vi "Find interstitial position.vi"(8 "Sublattice Index":i32, 9 "Interstitial Type":T3(ring), 10 "Suggested Location":dbl[](array[numeric])=[0.001, 6.609982847865, 13.218965695729999], 11 "Input Structure":T1={"Structure Name"="Gamma8_64atom Expanded to Box", "Lattice vector a"=[13.21796569573, 0.0, 0.0], "Lattice vector b"=[0.0, 13.21796569573, 0.0], "Lattice vector c"=[0.0, 0.0, 13.21796569573], "Atoms Array"=[{"Atom Name"="Cd", "Positions (Direct)"=array171x3[513 elements], "Positions (Cartesian)"=array171x3[513 elements]}, {"Atom Name"="Te", "Positions (Direct)"=array256x3[768 elements], "Positions (Cartesian)"=array256x3[768 elements]}], "# of atoms"=427}) -> (2 "Actual Position":dbl[](array[numeric])=[-1.6522457119662501, 8.261228559831249, 14.87021140769625])   [LabVIEW 2010]
uses:
  <vilib>/Analysis/_algsub.llb/Real Vector Norm.vi
  <vilib>/Analysis/NI_AALPro.lvlib
panel:
  out "Array 5":dbl[][](array[numeric])=[[4.672549508441724, 4.672549508441724, 4.672549508441726, 4.673256668714749, 4.6732566687147505, 4.673256668714748, 4.6732566687147505, 4.6732566687147505, 4.67325666871475, 4.673963721996005, 4.673963721996006, 4.673963721996005, 6.608482885695166, 6.608482885695166, 6.609482885689442, 6.609482885689441, 8.093501356604872, 8.093501356604872, 8.093909635782499, 8.093909635782499, 8.093909635782499, 8.093909635782499, 8.094317894366434, 8.094317894366432, 8.094317894366434, 8.094317894366434, 8.094726132359792, 8.09472613235979, 8.094726132359792, 8.094726132359792, 8.09513434976569, 8.09513434976569, 9.345806083535642, 9.346513217063759, 9.346513217063759, 9.346513217063759, 9.34722029709599, 10.449086969335582, 10.449086969335582, 10.449086969335582, 10.449086969335582, 10.449403211455978, 10.449403211455978, 10.449403211455978, 10.449403211455978, 10.45003566698613, 10.450035666986132, 10.450035666986132, 10.450035666986132, 10.450351880397623, 10.450351880397623, 10.450351880397623, 10.450351880397623, 11.446805432839044, 11.447382783106764, 12.363472966495479, 12.363472966495479, 12.363740242180455, 12.363740242180455, 12.364007512087667, 12.364007512087667, 12.364007512087667, 12.364274776217494, 12.364274776217494, 12.364274776217494, 12.364274776217494, 12.364274776217494, 12.364274776217494, 12.364542034570308, 12.364542034570308, 12.364542034570308, 12.364809287146482, 12.364809287146482, 12.365076533946393, 12.365076533946395, 13.217465714644366, 13.218465714642937, 14.019062667548008, 14.01906266754801, 14.019298379715233, 14.019298379715234, 14.0195340879194, 14.019769792160709, 14.019769792160709, 14.019769792160709, 14.02000549243936, 14.020241188755552, 14.02024118875555, 14.020476881109484, 14.020476881109484, 14.777464099713631, 14.777911326842537, 14.777911326842537, 14.77835854043732, 14.77835854043732, 14.77880574049921, 15.499012269911264, 15.499225475026416, 15.499225475026416, 15.499651876458502, 15.4996518764585, 15.49986507277568, 16.18822746580202, 16.188635719239674, 16.18863571923967, 16.189043962382037, 16.848881792586056, 16.84907791671063, 16.84907791671063, 16.84907791671063, 16.849274038552334, 16.849274038552334, 16.84947015811125, 16.849470158111252, 16.84966627538746, 16.84966627538746, 16.849666275387456, 16.84966627538746, 16.849862390381034, 16.849862390381034, 16.850058503092065, 16.850058503092065, 16.850254613520626, 16.850254613520622, 16.850254613520622, 16.850450721666792, 18.09871464894432, 18.09889722957616, 18.099079808366156, 18.099079808366156, 18.09926238531436, 18.09926238531436, 18.099627533685634, 18.099627533685634, 18.09981010510881, 18.09981010510881, 18.09999267469042, 18.10017524243052, 18.693026373944644, 19.267644542789487, 19.267987549118388, 19.26815904999305, 19.268159049993052, 19.268159049993052, 19.268502047163004, 19.268502047163004, 19.268502047163004, 19.268673543458373, 19.26901653147011, 19.826781895141632, 19.827115228474657, 20.36976655471307, 20.369928779363836, 20.37025322478959, 20.370253224789593, 20.370253224789593, 20.37025322478959, 20.370577665047854, 20.370739883239253, 21.415397772224, 21.41555207612973, 21.41555207612973, 21.41570637892368, 23.366000113979208, 23.366141536619267, 23.366282958403378, 23.36642437933155, 23.36656579940381, 24.282817476411132, 24.28308964193794], [4.121068592009394, 4.121068592009396, 4.121603126043498, 4.1216031260434995, 4.926194072761157, 4.9261940727611595, 5.616686189952471, 5.61668618995247, 5.617078399396615, 5.6170783993966165, 6.231480198063994, 5.61629395311869, 6.789868127999895, 7.7891381166692994, 7.789138116669298, 6.789543667070974, 7.306002937376851, 6.789868127999896, 8.242671674725111, 8.242671674725113, 7.788572438092881, 7.78885528251651, 8.673281849437187, 8.673281849437188, 9.083258983078276, 8.673535843492077, 8.673535843492076, 9.475746696494848, 9.47574669649485, 9.475979181314102, 9.475979181314104, 8.67277383901172, 9.475514205971507, 10.214936166974272, 10.214936166974274, 10.904736782714235, 9.082773903193985, 9.475049207810867, 10.214504829810819, 10.21450482981082, 9.475281709743651, 9.851940884561692, 10.904130700545782, 10.904130700545783, 11.233372335394707, 11.23337233539471, 11.552853748728355, 11.552853748728355, 11.553044435475528, 11.863920576351129, 11.553044435475526, 11.863920576351127, 11.552472365791504, 12.750981632607322, 11.232587861724038, 11.5520909702636, 11.863177798874412, 12.166131809314017, 12.166312883949994, 12.750636086798133, 12.750636086798133, 12.166493955891026, 12.750808860873262, 13.033146293985183, 13.309495784375729, 13.033146293985181, 13.309495784375729, 12.750981632607324, 13.580385110031902, 13.580385110031902, 13.84597564056925, 13.84597564056925, 13.8461347468455, 13.8461347468455, 13.309164739275896, 14.36212355005444, 13.308999213638101, 13.579736219180225, 14.105785805791598, 14.105785805791598, 14.612910408786753, 14.106098155620577, 14.860058287829462, 14.86005828782946, 14.860206536460197, 14.860354783611985, 15.342414924731075, 15.342558512555073, 15.577993369656815, 14.361356583700655, 15.34198415319593, 15.341984153195932, 15.342271335563247, 15.809643929002224, 16.263861920428326, 15.341840559996374, 15.57742769107951, 15.80936523661549, 16.705207092922233, 16.705207092922233, 16.921823947786486, 16.263184639667976, 16.705075217695192, 17.13531702235606, 17.55526852148856, 16.03753681002498, 16.704679585767526, 16.704679585767526, 16.485343319120254, 17.135059891331423, 17.135059891331423, 17.346309670416233, 17.346309670416233, 17.135317022356062, 17.555017541558783, 17.76114907877112, 17.76114907877112, 17.135445586421458, 17.9650382215233, 17.76139714593035, 17.965160847856563, 17.96528347335281, 18.166760470480675, 18.366027379531886, 18.366147328557506, 17.554515570934324, 17.964547707819758, 18.36542762265253, 18.365427622652533, 18.757742113038155, 18.757742113038155, 18.757977000635638, 18.95102838555922, 18.758094443331412, 19.331462290438033, 19.518955299633447, 19.51906816366124, 19.518616703634326, 18.757389776126885, 19.33100644902812, 19.518503836996, 19.88797484568549, 19.88797484568549, 19.704328959034704, 20.250923605296144, 20.42987230947458, 20.60737402688409, 20.78346583163942, 20.250706034368534, 20.957552569971597, 20.25048846110334, 20.606946409636635, 21.301975381695218, 20.783041837533364, 20.957447452744763, 21.301975381695218, 21.641222668030355, 21.808867468755267, 21.974732126453016, 22.13985170979759, 22.303650137269525, 22.46635242197059, 23.572912488272582, 23.726912670683017, 24.182847599331026, 24.482117462115625, 24.630433555487564, 24.77750622801834, 25.358484373325638, 0.0], [4.524587386078812, 5.09231998205977, 3.874966286339239, 4.524952541816038, 5.603111553104299, 6.50496138707789, 6.070806442471428, 5.092968857408524, 5.603406425376871, 6.505215379893139, 6.07053427389457, 7.660986458166829, 8.343679408145237, 7.661417786223605, 7.29572321537556, 8.0091972635348, 6.504707384344847, 8.664306600558447, 9.273072437942245, 8.664306600558449, 8.009609840002271, 8.6644972941253, 9.563106645654948, 9.844431954236441, 8.974221394458146, 8.009816120266752, 9.844599788361915, 10.118101441398835, 9.273606952723192, 9.563452185221488, 9.562761093602722, 10.117938144059453, 10.643887253154116, 11.145043715872097, 11.145340210668671, 9.272894259501733, 10.117611541473876, 10.897043574310901, 11.144747213187577, 9.562933871189628, 10.38408395483256, 11.624472396978694, 11.856989090555045, 10.897498434718967, 11.857267782941785, 12.30912112407838, 11.624756663731397, 11.857407126678797, 12.309255352727742, 11.145340210668671, 11.857407126678797, 12.528674536829765, 13.37212106489996, 11.856710391617629, 12.308584194842918, 12.744575824396993, 13.166012172053, 12.957135069939262, 13.166137664709101, 13.774130693526065, 12.528806413271395, 13.574614140679618, 13.971034773386775, 14.16508540124641, 13.166263156169087, 13.971034773386775, 13.166388646432988, 13.971153035115119, 14.356628458710277, 14.35674354416327, 14.165318683582521, 13.971389555568704, 13.774610496418132, 14.164852115068351, 14.916285749111236, 14.16473547053853, 14.356168107672538, 14.731684587922098, 15.097754613480275, 15.45526325984557, 14.73190889806441, 15.8046869786592, 15.27771694780128, 15.63111010771154, 15.277933241115514, 15.976688369673775, 15.631321511063923, 15.805000600052866, 15.277392502088265, 15.976378118566092, 16.314543247000234, 15.976584953307304, 16.646038384911055, 16.646236898914424, 16.31444197227772, 16.481024032009135, 16.809039732075895, 17.289589961986348, 17.446769123222808, 17.44686382506795, 17.28930327050073, 17.60245096948259, 17.90993980179392, 18.212419286233594, 16.808744844283712, 17.446390310701666, 17.602169373652973, 17.44639031070167, 17.909755294839574, 18.061538320598714, 17.75676793301744, 18.361430624238494, 17.909939801793918, 18.509599424233063, 18.65650295824463, 18.361520608602852, 17.60254483375806, 18.802346633009304, 18.361700576008616, 18.65668008017071, 18.361790559050036, 18.65676864050317, 18.80252238107122, 18.509956477832805, 18.36116066849946, 18.946631698736383, 18.946718903783477, 19.37414908003062, 19.514630123374026, 19.654023014068105, 19.514799456692987, 19.792601178364315, 19.233071485218513, 20.066639715409647, 20.066722053177486, 19.792851610620946, 20.470537751643775, 19.65377081282996, 20.33657972898106, 20.470457038133002, 20.470457038133002, 20.866698509977905, 20.33682346256355, 21.126887590461724, 21.126887590461724, 21.255787812660607, 21.12712220663944, 21.25555461667795, 21.763376075120195, 21.255399151268165, 21.637347178603495, 22.13641183778336, 21.637499899717355, 21.88837740631114, 22.01274397403771, 22.38184535746878, 22.381919178146244, 22.983390678019713, 23.101934623215634, 23.219802219673422, 23.33714531380384, 24.59005058073211, 24.700885082114148, 25.139139911160846, 25.247564075565105, 25.35552460562809, 25.782397904268457, 26.202633032169903, 0.0, 0.0]]
  out "Array 4":dbl[][](array[numeric])=[[0.5476079792120737, 0.547607979212074, 0.5476079792120737, 0.5473669639053449, 0.5473669639053448, 0.547366963905345, 0.5473669639053449, 0.5473669639053448, 0.5473669639053448, 0.5474874317712398, 0.5474874317712399, 0.5474874317712396, 0.4166189217542727, 0.41661892175427284, 0.4165658301235803, 0.4165658301235802, 1.0485123471873823, 1.0485123471873823, 0.3494728260287518, 0.34947282602875185, 0.3494728260287518, 0.3494728260287518, 1.0476668985331294, 0.3494101580745812, 0.3494101580745813, 1.047666898533129, 1.0485123471873823, 1.048512347187383, 1.0485123471873823, 1.0485123471873823, 0.3494728260287518, 0.34947282602875185, 0.5474874317712397, 0.547366963905345, 0.5473669639053449, 0.5473669639053449, 0.5476079792120738, 0.4165658301235802, 0.41656583012358017, 0.4165658301235804, 0.4165658301235802, 0.4166189217542728, 0.4166189217542727, 0.4166189217542727, 0.4166189217542728, 0.41656583012358017, 0.41656583012358017, 0.4165658301235802, 0.41656583012358006, 0.41661892175427284, 0.4166189217542727, 0.4166189217542727, 0.4166189217542726, 0.3494728260287518, 1.0485123471873827, 0.5473669639053449, 0.5473669639053451, 0.5474874317712397, 0.5474874317712396, 0.5476079792120739, 0.5476079792120737, 0.5476079792120737, 0.5473669639053449, 0.5473669639053448, 0.5473669639053448, 0.5473669639053451, 0.30695887398929206, 0.5473669639053451, 0.5474874317712398, 0.5474874317712396, 0.5474874317712397, 0.5476079792120739, 0.5476079792120737, 0.30695887398929206, 0.30695887398929206, 0.4165658301235802, 0.4166189217542728, 0.3494101580745812, 0.3494101580745813, 1.0485123471873825, 1.048512347187382, 0.34947282602875185, 0.3495041726531689, 0.34950417265316897, 0.34950417265316885, 1.0485123471873818, 0.3494728260287518, 0.34947282602875185, 0.2542774918608737, 0.3495041726531689, 0.5473669639053448, 0.5476079792120739, 0.5476079792120742, 0.5474874317712396, 0.5474874317712399, 0.30695887398929206, 0.4165658301235803, 0.4166189217542727, 0.4166189217542727, 0.4165658301235802, 0.4165658301235803, 0.4166189217542727, 1.0485123471873825, 1.047666898533129, 0.3494101580745812, 0.3494728260287518, 0.3068739535103656, 0.5473669639053448, 0.5473669639053448, 0.5473669639053448, 0.5474874317712397, 0.5474874317712399, 0.5476079792120737, 0.5476079792120738, 0.5473669639053448, 0.5473669639053451, 0.30695887398929217, 0.30695887398929206, 0.3069164049386094, 0.3069164049386095, 0.5476079792120738, 0.5476079792120742, 0.30695887398929217, 0.30695887398929217, 0.306958873989292, 0.23641690930736067, 0.34937883673726944, 1.047666898533129, 1.0485123471873825, 1.048512347187382, 0.3494728260287518, 0.34947282602875185, 1.048512347187383, 1.0485123471873827, 0.3494728260287518, 0.34947282602875185, 0.2542774918608737, 0.20968219392944848, 0.3069588739892921, 0.4164597077251133, 0.41656583012358017, 0.4164597077251134, 0.4166189217542727, 0.41661892175427284, 0.41656583012358017, 0.41656583012358045, 0.2768971596369435, 0.2769127510076522, 0.22185040368770584, 0.3494728260287518, 0.254253349262326, 0.5473669639053448, 0.5474874317712397, 0.23640720642010601, 0.547366963905345, 0.5473669639053452, 0.23640720642010596, 0.23639750472741433, 0.23640720642010601, 0.34947282602875174, 0.3494101580745812, 0.2542774918608737, 0.25425334926232607, 0.3069164049386094, 0.3068739535103656, 0.23640720642010607, 0.1993015788370914, 0.19930739241282994, 0.25426541970196903, 0.18250028210459257], [0.8561932504079697, 0.8561932504079697, 0.38283173606959353, 0.38283173606959353, 0.4280318477924466, 0.4280318477924465, 0.4942735398142433, 0.49427353981424343, 0.4941239710797636, 0.4941239710797636, 0.3494865422516429, 0.4942236684792082, 0.8561932504079699, 0.49412397107976336, 0.49412397107976347, 0.8559341113720182, 2309.4010767618342, 0.38280856217615494, 0.6053284338785394, 0.6053284338785391, 0.49422366847920796, 0.4940741450001373, 0.38283173606959353, 0.38283173606959353, 0.4280318477924465, 0.855675207490044, 0.8556752074900444, 0.4941239710797636, 0.49412397107976347, 0.4941738122369185, 0.4941738122369186, 0.8559341113720185, 0.4940741450001371, 0.38283173606959353, 0.38283173606959353, 0.4941738122369186, 0.4279670777316935, 0.4941738122369187, 0.8559341113720187, 0.8559341113720187, 0.49422366847920807, 0.34945128322800595, 0.4942236684792083, 0.49422366847920807, 0.6051452780610137, 0.6051452780610137, 0.3827622270115112, 0.3827622270115112, 0.8559341113720186, 0.4279670777316935, 0.8559341113720186, 0.4279670777316935, 0.38280856217615494, 0.8556752074900443, 0.6051452780610139, 0.8556752074900441, 0.42796707773169335, 0.49417381223691836, 0.49422366847920796, 0.38280856217615494, 0.38280856217615494, 0.4940741450001373, 0.38283173606959353, 0.30264132246286574, 0.4940741450001373, 0.30264132246286574, 0.4940741450001374, 0.855675207490044, 0.6051452780610139, 0.6051452780610139, 0.8559341113720187, 0.8559341113720182, 0.38280856217615494, 0.38280856217615494, 0.4941738122369187, 0.4941738122369186, 0.4941239710797636, 0.6051452780610138, 0.4279670777316935, 0.4279670777316935, 0.349451283228006, 0.4280318477924465, 0.38283173606959353, 0.38283173606959353, 0.3827622270115112, 0.8559341113720186, 0.4941738122369187, 0.4942236684792083, 0.6053284338785394, 0.49412397107976347, 0.4942236684792083, 0.4942236684792082, 0.49412397107976336, 0.3827622270115112, 0.4942236684792083, 0.49417381223691836, 0.6053284338785391, 0.38280856217615494, 0.8556752074900441, 0.8556752074900447, 2309.4010767618342, 0.4941738122369185, 0.38283173606959353, 0.4940741450001373, 0.8559341113720189, 0.4279023370651891, 0.3827622270115112, 0.3827622270115112, 0.349416034873861, 0.4941738122369187, 0.4941738122369187, 0.6053284338785394, 0.6053284338785394, 0.4942735398142433, 0.38283173606959353, 0.4280318477924466, 0.4280318477924465, 0.4941239710797636, 0.4941239710797636, 0.4279670777316935, 0.4941738122369187, 0.49422366847920807, 0.349451283228006, 0.8561932504079697, 0.38283173606959353, 0.38273906573776, 0.4941239710797636, 0.8559341113720189, 0.8559341113720185, 0.49422366847920807, 0.4942236684792082, 0.49412397107976347, 0.6051452780610139, 0.49417381223691836, 0.4279670777316935, 0.49422366847920807, 0.3235406796961882, 0.49427353981424343, 0.32348473632136465, 0.4279670777316935, 0.49422366847920807, 0.8561932504079699, 0.8561932504079699, 0.34948654225164283, 0.4941239710797636, 0.6051452780610138, 0.8559341113720187, 0.4280318477924465, 0.4942236684792082, 0.4941239710797636, 0.4941239710797636, 0.8559341113720185, 0.38283173606959353, 0.4280318477924464, 0.4940741450001373, 0.38283173606959353, 0.4941738122369185, 0.6053284338785391, 0.8561932504079699, 0.4280318477924465, 0.49427353981424343, 0.3494865422516429, 0.4941738122369187, 0.34945128322800595, 0.4942735398142433, 0.3827622270115112, 0.42796707773169335, 0.49422366847920807, 0.32355467007556094, 0.0], [0.5115804251230851, 0.5824808304777034, 0.33219352288401144, 0.5114389056756381, 0.3940200961906628, 0.4615602383379139, 0.4238058809752943, 0.5823241605883408, 0.3939554262004827, 0.46145629586343273, 0.4237857592774801, 0.6944091253052345, 0.4614562958634326, 0.694143717868172, 0.5824285931318084, 0.912579492565525, 0.33218383231913956, 0.5115804251230849, 0.6944091253052346, 0.5115804251230851, 0.4237053011371849, 0.5114389056756379, 0.4238058809752943, 0.46156023833791365, 0.5823241605883406, 0.9121779329760806, 0.46145629586343256, 0.34947596486447613, 0.6942321531975371, 0.42374552447850033, 0.9125794925655242, 0.5114389056756379, 0.3940200961906628, 0.46156023833791365, 0.46148227489852917, 0.3939877572149216, 0.5115450342478336, 0.9125794925655255, 1.7482263996378062, 0.42378575927747997, 0.3697306291319899, 0.5824808304777032, 0.6944091253052349, 0.9121779329760806, 0.6941437178681721, 0.46145629586343256, 0.5823241605883405, 0.6942321531975371, 0.46148227489852917, 1.746815611858634, 0.6942321531975371, 0.5115804251230848, 0.46145629586343256, 0.6942321531975368, 1.7468156118586362, 0.5824285931318085, 0.9125794925655252, 0.39400392570742504, 0.42378575927748025, 0.5824808304777033, 0.5114389056756379, 0.5114389056756378, 0.3940200961906627, 0.42380588097529426, 0.4237053011371851, 0.3940200961906629, 0.9121779329760801, 0.3939554262004827, 0.4614562958634326, 0.4614822748985293, 0.4237455244785002, 0.3939877572149216, 0.5824285931318082, 0.912579492565525, 0.694232153197537, 0.9123786464948287, 1.7468156118586369, 0.5824285931318082, 0.9125794925655252, 0.511580425123085, 0.5822719653781748, 0.39402009619066275, 0.33219352288401144, 0.5823241605883405, 1.746815611858634, 0.4237455244785004, 0.5824285931318082, 0.3939877572149215, 1.7468156118586322, 0.42378575927748013, 0.511580425123085, 0.91217793297608, 0.3939554262004827, 0.3939877572149216, 0.5115450342478336, 0.3697306291319898, 0.4237857592774801, 0.5823241605883407, 0.6941437178681721, 0.6942321531975367, 0.5824285931318082, 0.4237053011371851, 0.5114389056756379, 0.6942321531975366, 0.9121779329760806, 0.6942321531975374, 0.9123786464948292, 0.6942321531975371, 0.5115450342478336, 0.5824285931318088, 0.33218383231913956, 0.4237857592774801, 0.5114389056756378, 0.33219352288401144, 0.5114389056756381, 0.4237053011371849, 0.9121779329760801, 0.5823241605883409, 0.912378646494829, 0.511509650716535, 0.9125794925655255, 0.5115450342478336, 0.5824285931318084, 0.33218383231913956, 0.9121779329760811, 0.6942321531975372, 0.39398775721492163, 0.5115450342478336, 0.36973062913199, 0.39400392570742504, 0.5823241605883406, 0.42372541137597447, 1.7468156118586353, 0.5115096507165352, 0.5115450342478337, 0.42378575927748025, 0.4237053011371851, 0.6941437178681722, 0.39398775721492146, 0.4237857592774801, 0.4237857592774801, 0.36973062913198984, 0.6941437178681722, 0.42372541137597447, 0.9121779329760803, 1.7468156118586347, 0.42378575927748013, 0.3321838323191395, 0.9121779329760801, 0.4614822748985293, 0.3939877572149215, 0.582271965378175, 0.3940200961906627, 0.3321935228840115, 0.511438905675638, 0.9123786464948292, 0.912579492565525, 0.4237857592774801, 0.3321935228840115, 0.5114389056756382, 0.582324160588341, 0.3939877572149215, 0.4237857592774801, 0.39402009619066275, 0.9121779329760809, 1.7468156118586369, 0.4237857592774801, 0.6941437178681724, 0.0, 0.0]]
  out "Array 3":dbl[][](array[numeric])=[[1.9547268638345616, 2.8620737470709985, 3.5435417267010227, 4.113946207379072, 4.114267491346153, 4.614370902468288, 4.614657345750077, 5.065859043343244, 5.479794675188183, 5.864811600602199, 6.226064610883467, 7.202091391883803], [1.7167946955093463, 3.418443867660097, 3.418443867660097, 4.006367470857006, 4.006367470857007, 4.519014199249397, 4.978625429595594, 4.978625429595595, 4.978890916796135, 5.789856822486257, 5.789856822486257, 6.500831983269877], [3.0102934919328925, 3.010732552172754, 3.0107325521727546, 3.6646599209082016, 3.6646599209082025, 3.665020590535618, 5.151307815891239, 5.5588842449956095, 5.55888424499561, 6.955045345834196, 6.955045345834196, 6.955235391828881], [1.955267753201033, 2.861519495286735, 3.5434671227829164, 4.113881947574676, 4.114203236559899, 4.614600058516157, 4.614600058516158, 5.065545926675186, 5.864766524929215, 6.567436124440425, 6.891957826114611, 7.499163761830803], [2.5379416168562856, 2.5384623778402253, 3.2881083729171117, 3.8957513405305857, 4.420943783354774, 4.421242758402029, 4.421242758402029, 4.890052081923117, 5.713872611512734, 6.084094480605371, 6.084311731171563, 6.433045241351105], [2.166564441514756, 3.010732552172755, 3.010732552172756, 3.665020590535619, 4.708021154645086, 4.708021154645086, 5.151051215132988, 5.151051215132988, 5.15130781589124, 5.5588842449956095, 5.55888424499561, 5.938998490548465], [2.3595708433746223, 2.360130962053328, 3.7823205859257243, 3.782320585925725, 4.3210150254211985, 4.321015025421199, 5.235160141446535, 5.235160141446536, 5.235412619816098, 6.011874297027946, 6.011874297027946, 6.6993288479577675], [1.7172565860734128, 3.4179024921650596, 3.4182891976963075, 4.0062354991045535, 4.006565420335059, 4.518897199069925, 4.9785192307512744, 4.9785192307512744, 6.500547318827066, 6.500547318827066, 7.14092755186499, 7.141112650989596], [2.5383582341904414, 2.5383582341904423, 3.2876259459191286, 3.896022764532719, 4.420883985919037, 4.420883985919037, 4.421182965009993, 5.713826345100761, 5.713826345100762, 6.433209615097385, 6.763978695041821, 6.763978695041822], [2.1670524575439933, 3.0102056722001067, 3.0106447452472453, 3.6649484594496307, 4.707965003476324, 4.708245752623474, 5.150999893447406, 5.150999893447408, 5.938731409903124, 5.938731409903126, 6.295744291766251, 6.295954239068649], [2.3596828777468075, 3.152137165776393, 3.152556471343213, 3.7820410019202884, 3.7823904786980087, 4.32138208929536, 4.799954686961217, 5.235463114028928, 5.636958031913642, 6.364827311893895, 6.699171003830835, 6.6993683084084115], [1.4400732414920958, 3.288188770535453, 3.8961584694430518, 3.8961584694430518, 4.421003579981707, 4.421003579981707, 4.890106142257899, 4.890106142257899, 5.31798867156426, 5.31798867156426, 5.714150202117751, 6.433291800395586], [2.167052457543994, 3.0102056722001067, 3.0106447452472445, 3.66494845944963, 4.707965003476324, 4.708245752623474, 5.150999893447406, 5.150999893447408, 5.55907446647117, 5.9387314099031245, 5.938731409903125, 6.295744291766251], [1.4406238567874132, 3.2876259459191286, 3.896022764532718, 3.8960227645327183, 4.420883985919039, 4.420883985919039, 4.890268319676531, 5.713826345100761, 5.713826345100761, 6.76397869504182, 6.76397869504182, 7.0796833833481685], [1.7169486728370351, 3.4181345207337306, 3.4181345207337324, 4.006763360033648, 4.0067633600336485, 4.978678528168266, 4.978678528168268, 4.978944012537486, 5.399791561562377, 6.1555532791013885, 6.155553279101389, 7.141223708161447], [1.0957949506280387, 3.782110899859237, 3.7824603701788044, 4.321137383510436, 4.321137383510436, 4.321443263576482, 4.800285127848961, 5.235261134255497, 5.235261134255498, 5.637004929231793, 5.637239409970335, 7.017829427869573], [3.0103813091037743, 3.0103813091037743, 3.010381309103776, 3.665092720202024, 3.6650927202020243, 3.6650927202020247, 5.558931800974737, 5.558931800974738, 5.939043002821646, 7.2623033473943455, 7.2623033473943455, 7.5572189945145585], [1.9547268638345625, 2.862073747070998, 3.5435417267010223, 4.113946207379072, 4.114267491346153, 4.614370902468288, 4.614657345750078, 5.479794675188184, 5.864811600602199, 5.865036973770693, 6.226064610883468, 7.202091391883803], [1.4400732414920956, 3.2881887705354536, 3.8961584694430518, 3.896158469443052, 4.421003579981706, 4.421003579981707, 4.890106142257899, 4.890106142257899, 5.31798867156426, 5.31798867156426, 5.714150202117751, 5.714150202117753], [1.9547268638345618, 2.8620737470709994, 3.5435417267010214, 4.113946207379071, 4.114267491346154, 4.614370902468289, 4.614657345750079, 5.065859043343244, 5.479794675188184, 5.8648116006021995, 5.865036973770694, 6.226064610883468], [2.3601309620533297, 3.1520532979695948, 3.1520532979695948, 3.782320585925725, 3.7823205859257256, 4.321015025421198, 4.799899611268254, 5.235412619816098, 6.364785777353597, 6.364993447344765, 6.699131542217993, 7.322164589560574], [1.955267753201034, 2.861519495286734, 3.543467122782916, 4.113881947574677, 4.114203236559898, 4.614600058516157, 5.065545926675185, 5.479987642023664, 5.864766524929215, 6.567436124440424, 6.89195782611461, 7.499163761830803], [2.3595708433746223, 2.3601309620533284, 3.7823205859257247, 3.782320585925725, 4.3210150254211985, 4.3210150254211985, 5.235160141446535, 5.235160141446536, 5.235412619816097, 5.235412619816097, 6.011874297027946, 6.011874297027946], [2.166564441514757, 3.0107325521727546, 3.0107325521727555, 3.665020590535619, 4.708021154645086, 4.708021154645086, 5.151051215132988, 5.151051215132989, 5.55888424499561, 5.558884244995611, 5.938998490548465, 5.938998490548466], [1.7172565860734135, 3.4179024921650596, 3.4182891976963075, 4.006235499104553, 4.006565420335059, 4.518897199069925, 4.978519230751274, 4.9785192307512744, 5.789993797990992, 6.500547318827066, 6.500547318827066, 7.14092755186499], [1.0962773422257543, 3.781901202166781, 3.781901202166783, 4.320953845077257, 4.321259738135057, 4.3212597381350575, 4.800119910248538, 5.636864236106813, 6.364744242542257, 7.322128485487463, 7.614553892797943, 7.8963244619126955], [2.1670524575439942, 3.0102056722001063, 3.010644745247245, 3.6649484594496307, 4.707965003476324, 5.150999893447406, 5.150999893447407, 5.55907446647117, 5.9387314099031245, 5.938731409903125, 6.295744291766251, 6.295954239068649], [2.861427109551845, 2.8618890084029047, 2.8618890084029056, 2.861889008402906, 5.479698189222204, 5.479698189222204, 5.479698189222205, 5.479698189222205, 5.479698189222205, 5.479698189222205, 5.479939400951825, 5.479939400951825], [1.4404403417417915, 3.2879475717827327, 3.8956156214377966, 3.895954910304962, 4.421123170809281, 4.889943959460572, 5.317839538290181, 5.713780078314153, 6.432963052902951, 6.76393961152462, 6.764135026852361, 7.07945933646696], [2.3599069305349967, 2.3599069305349976, 3.7818313003520827, 3.7821807965064096, 4.321198561255806, 5.235059146689258, 5.235059146689258, 6.011786350662306, 6.011786350662306, 6.012006214164183, 6.699052618294945, 6.699052618294945], [1.0957949506280396, 3.782110899859236, 3.7824603701788044, 4.321137383510435, 4.321137383510437, 4.321443263576482, 4.800285127848962, 5.235261134255497, 5.235261134255499, 5.637004929231793, 5.637239409970335, 6.365076513444079], [1.955267753201034, 2.861519495286735, 3.543467122782915, 4.113881947574675, 4.1142032365598995, 4.6146000585161575, 4.614600058516158, 5.065545926675186, 5.479987642023664, 5.864766524929215, 6.567436124440425, 6.891957826114611], [2.5379416168562856, 2.538462377840225, 3.288108372917112, 3.8957513405305866, 4.420943783354774, 4.421242758402028, 4.890052081923118, 5.713872611512733, 6.084094480605371, 6.084311731171562, 6.433045241351105, 6.764213191402724], [2.166564441514757, 3.010732552172755, 3.010732552172755, 3.6650205905356184, 4.708021154645086, 4.7080211546450865, 5.151051215132988, 5.151051215132988, 5.15130781589124, 5.55888424499561, 5.55888424499561, 5.938998490548465], [2.1669304638404157, 3.0105569357607256, 3.010556935760726, 3.6645156431178245, 5.151205177121809, 5.558789131816816, 5.558789131816817, 5.938686895294458, 5.938686895294458, 5.938909465001236, 6.295702301465619, 6.29570230146562], [2.5381499340714204, 2.538149934071421, 3.2878671682664047, 3.8962263201257508, 4.421362342760207, 4.421362342760208, 4.890160201995049, 5.713965143212813, 6.084398629226024, 6.7640959442384565, 7.07960870184225, 7.381826900752755], [1.9548621002066446, 2.861704257808922, 3.543989317229699, 4.114010466179742, 4.114010466179744, 4.6147146322728325, 5.065911227573018, 5.480084122893345, 5.864856675928745, 5.8648566759287455, 6.567516630040667, 6.567717889723938], [1.095794950628038, 3.782110899859237, 3.782460370178805, 4.321137383510435, 4.321137383510437, 4.321443263576482, 4.800285127848962, 5.235261134255497, 5.235261134255498, 5.637004929231793, 6.365076513444079, 7.017829427869573], [0.5720082937811589, 4.219158541065158, 4.219158541065159, 4.219158541065159, 4.708133454973564, 4.708133454973564, 4.708133454973565, 4.708133454973565, 4.708133454973566, 4.708133454973566, 6.296080204089681, 6.296080204089682], [2.359682877746808, 3.152137165776393, 3.152556471343213, 3.7820410019202884, 3.782390478698009, 4.321382089295359, 4.799954686961217, 6.012138128405919, 6.364827311893896, 7.0176034062139205, 7.01779175809915, 7.6146233277543], [2.704671783205201, 2.7046717832052014, 2.7051604477379074, 4.006367470857006, 4.518721693120581, 4.519014199249398, 4.519014199249399, 5.399742604022198, 6.1555103324767515, 6.15572506260369, 6.500628652797005, 7.141001592090578], [1.716794695509347, 3.418443867660096, 3.418443867660097, 4.006367470857005, 4.006367470857006, 4.519014199249398, 4.978625429595593, 4.978625429595595, 5.789856822486258, 5.789856822486258, 6.500831983269877, 6.500831983269878], [1.440073241492095, 3.2881887705354536, 3.896158469443052, 3.8961584694430527, 4.421003579981705, 4.421003579981706, 4.890106142257899, 4.890106142257899, 5.31798867156426, 5.31798867156426, 5.714150202117752, 6.433291800395587], [1.0962773422257543, 3.7819012021667815, 3.781901202166783, 4.320953845077257, 4.321259738135057, 4.800119910248538, 5.235362125116258, 5.636864236106813, 6.364744242542257, 7.322128485487463, 7.614553892797943, 7.8963244619126955], [1.440623856787413, 3.287625945919129, 3.8960227645327183, 3.8960227645327183, 4.420883985919039, 4.420883985919039, 4.890268319676531, 4.890268319676531, 5.713826345100761, 5.713826345100762, 6.76397869504182, 6.763978695041821], [2.1670524575439942, 3.0102056722001067, 3.010644745247244, 3.6649484594496307, 4.707965003476324, 4.708245752623473, 5.150999893447407, 5.150999893447407, 5.55907446647117, 5.938731409903125, 5.938731409903125, 6.295744291766251], [1.717256586073414, 3.417902492165059, 3.418289197696307, 4.0062354991045535, 4.518897199069926, 4.978519230751274, 4.9785192307512744, 5.789993797990992, 6.500547318827066, 6.500547318827066, 7.14092755186499, 7.141112650989595], [1.4404403417417915, 3.2879475717827327, 3.895615621437797, 3.8959549103049618, 4.421123170809282, 4.889943959460573, 5.317839538290181, 5.318088091423596, 5.713780078314154, 6.432963052902951, 6.763939611524621, 7.07945933646696], [2.1669304638404157, 3.0105569357607256, 3.010556935760726, 3.664515643117825, 5.151205177121809, 5.151205177121809, 5.558789131816817, 5.558789131816817, 5.938686895294458, 5.938686895294459, 6.295702301465619, 6.29570230146562], [0.5724702671600166, 4.218594591447799, 4.218907906097472, 4.218907906097472, 4.707908851637849, 4.707908851637849, 4.708189604133328, 6.29570230146562, 6.29570230146562, 7.556939141082784, 7.556939141082784, 7.557114050692112], [1.4404403417417915, 3.2879475717827327, 3.895615621437797, 3.895954910304962, 4.889943959460573, 5.317839538290181, 5.318088091423596, 5.713780078314153, 6.432963052902951, 6.76393961152462, 6.764135026852361, 7.07945933646696], [1.954726863834563, 2.8620737470709985, 3.5435417267010214, 4.113946207379071, 4.114267491346154, 4.614370902468288, 4.614657345750079, 5.065859043343244, 5.479794675188184, 5.8648116006021995, 5.865036973770693, 6.226064610883469], [2.1670524575439942, 3.0102056722001067, 3.0106447452472445, 3.66494845944963, 4.707965003476324, 5.150999893447406, 5.150999893447408, 5.55907446647117, 5.9387314099031245, 5.938731409903125, 6.295744291766251, 6.2959542390686485], [1.440440341741792, 3.2879475717827322, 3.895954910304963, 4.421123170809281, 4.421422133726416, 4.890484547868772, 5.318088091423597, 5.714011408500935, 5.714242729322756, 5.714242729322757, 6.084224831875973, 7.079832743996675], [0.5724702671600158, 4.218907906097473, 4.218907906097475, 4.708189604133327, 4.708189604133329, 4.708470339888346, 4.708470339888347, 5.151205177121807, 5.151205177121808, 5.15146177021102, 6.296122191869992, 6.955349416933166], [1.716948672837035, 3.4181345207337306, 3.4181345207337315, 3.4185212000177447, 4.978678528168267, 4.978678528168267, 4.978944012537486, 4.978944012537487, 5.7901307702553355, 5.790130770255336, 6.1555532791013885, 6.1555532791013885], [1.0957949506280384, 3.7821108998592363, 3.7824603701788058, 4.321137383510435, 4.321137383510436, 4.321443263576483, 4.800285127848962, 5.235261134255498, 5.235261134255498, 5.637004929231793, 5.637239409970336, 6.365076513444079], [2.5380457776011314, 2.5385665172175567, 3.2877867627837887, 3.2877867627837896, 4.890376434967719, 4.8903764349677195, 5.317988671564261, 5.317988671564262, 5.318237217727783, 5.318237217727784, 6.7640568613987355, 6.764056861398736], [2.3596828777468066, 3.1521371657763946, 3.152556471343214, 3.7820410019202866, 3.782390478698008, 4.799954686961218, 5.235463114028927, 5.6369580319136405, 6.364827311893895, 6.699171003830835, 6.699368308408412, 7.32238121026089], [1.7167946955093467, 3.4184438676600966, 3.4184438676600974, 4.006367470857005, 4.006367470857006, 4.519014199249398, 4.978625429595593, 4.978625429595595, 4.978890916796135, 5.789856822486258, 5.789856822486258, 6.500831983269878], [1.9552677532010339, 2.8615194952867355, 3.543467122782915, 4.113881947574676, 4.1142032365598995, 4.6146000585161575, 5.065545926675186, 5.479987642023664, 5.864991899829825, 6.567436124440425, 7.201871153060142, 7.784772248560299], [1.9552677532010343, 2.861519495286735, 3.5434671227829146, 4.113881947574676, 4.114203236559899, 4.6146000585161575, 4.614600058516158, 5.065545926675185, 5.479987642023664, 5.864766524929216, 6.567436124440424, 6.891957826114612], [2.5379416168562865, 2.538462377840225, 3.288108372917112, 3.895751340530586, 4.420943783354774, 4.421242758402028, 4.421242758402029, 4.890052081923117, 5.713872611512734, 6.084094480605372, 6.084311731171562, 6.433045241351106], [2.3595708433746228, 2.3601309620533275, 3.782320585925725, 3.7823205859257256, 4.321015025421198, 4.321015025421198, 5.235160141446536, 5.235160141446536, 5.235412619816097, 6.011874297027947, 6.011874297027947, 6.699328847957769], [2.360130962053329, 3.152053297969595, 3.152053297969597, 3.7823205859257243, 4.321015025421197, 4.799899611268255, 5.235412619816096, 6.364785777353596, 6.364993447344764, 6.699131542217993, 7.322164589560574, 7.614762195767592], [2.537941616856285, 2.5384623778402253, 3.2881083729171126, 3.895751340530585, 4.420943783354774, 4.421242758402029, 4.890052081923117, 5.713872611512734, 6.084094480605371, 6.084311731171563, 6.433045241351106, 6.764213191402725], [1.096277342225755, 3.781901202166782, 3.781901202166782, 4.320953845077256, 4.321259738135058, 4.321259738135058, 4.800119910248539, 5.235362125116259, 5.636864236106814, 6.364744242542257, 7.322128485487464, 7.614553892797944], [2.5383582341904414, 2.5383582341904427, 3.2876259459191286, 4.420883985919037, 4.420883985919037, 4.421182965009993, 5.713826345100761, 5.713826345100762, 6.433209615097384, 6.433209615097385, 6.763978695041821, 6.763978695041822], [2.167052457543994, 3.0102056722001076, 3.0106447452472445, 3.66494845944963, 4.707965003476324, 4.708245752623474, 5.150999893447406, 5.150999893447408, 5.938731409903125, 5.938731409903125, 6.295744291766252, 6.2959542390686485], [2.166930463840415, 3.010556935760726, 3.0105569357607265, 3.6645156431178245, 5.151205177121808, 5.558789131816816, 5.558789131816816, 5.938686895294458, 5.938686895294459, 5.938909465001236, 6.29570230146562, 6.29570230146562], [2.359906930534997, 2.3599069305349976, 3.7818313003520823, 3.7821807965064105, 5.235059146689257, 5.235059146689258, 6.011786350662305, 6.011786350662306, 6.012006214164183, 6.012006214164183, 6.699052618294945, 6.699052618294945], [2.5381499340714204, 2.5381499340714213, 3.287867168266403, 4.4207643886210155, 4.89016020199505, 5.713965143212812, 6.083964126541941, 6.083964126541942, 6.432921958285101, 6.432921958285102, 6.763900527781585, 6.763900527781585], [1.7169486728370358, 3.4181345207337306, 3.4181345207337306, 4.518487674583966, 4.978678528168267, 5.78967418343894, 5.78967418343894, 6.500465983839474, 6.500465983839474, 6.500669319400369, 7.140853510871712, 7.140853510871712], [1.0957949506280387, 3.782110899859236, 3.7824603701788044, 4.321137383510434, 4.321137383510437, 4.321443263576482, 4.800285127848962, 5.235261134255497, 5.235261134255499, 5.637004929231793, 6.3650765134440785, 7.017829427869574], [1.4404403417417917, 3.2879475717827322, 3.895615621437797, 3.8959549103049618, 4.421123170809282, 4.889943959460573, 5.317839538290181, 5.318088091423596, 5.713780078314154, 6.432963052902951, 6.76393961152462, 7.07945933646696], [1.0960361729659003, 3.78218079650641, 3.782180796506411, 4.321504436991634, 4.800064836451338, 4.80006483645134, 5.23556410099362, 5.235564100993621, 5.637051826159785, 5.6370518261597855, 6.365118046087225, 6.365118046087226], [0.5724702671600156, 4.218907906097472, 4.218907906097474, 4.708189604133327, 4.708189604133329, 4.708470339888346, 4.708470339888346, 5.151205177121808, 5.151205177121808, 5.15146177021102, 6.955349416933166, 6.955349416933167], [1.7169486728370358, 3.4181345207337297, 3.4181345207337315, 4.006763360033647, 4.006763360033648, 4.978678528168266, 4.978678528168268, 5.399791561562377, 6.155553279101389, 6.15555327910139, 7.141223708161448, 7.141223708161449], [1.0957949506280384, 3.7821108998592363, 3.782460370178805, 4.321137383510434, 4.321137383510437, 4.321443263576483, 4.800285127848962, 5.235261134255497, 5.235261134255499, 5.637004929231793, 5.637239409970336, 7.017829427869574], [1.9547268638345623, 2.862073747070999, 3.5435417267010205, 4.113946207379071, 4.114267491346154, 4.614370902468288, 4.614657345750079, 5.4797946751881845, 5.8648116006021995, 5.865036973770694, 6.226064610883469, 7.202091391883804], [1.7174105219895286, 3.4179798367714156, 3.4179798367714156, 3.417979836771416, 4.978837820488555, 4.978837820488555, 4.978837820488556, 4.978837820488556, 5.789811163264552, 5.789811163264553, 7.440513453247007, 7.440513453247008], [2.537941616856286, 2.538462377840225, 3.2881083729171126, 3.895751340530585, 4.420943783354774, 4.421242758402029, 4.421242758402029, 4.890052081923117, 5.713872611512734, 6.084094480605372, 6.433045241351107, 6.764213191402725], [3.0102934919328925, 3.010732552172754, 3.010732552172755, 3.6646599209082007, 3.6646599209082025, 5.15130781589124, 5.558884244995609, 5.55888424499561, 6.955045345834196, 6.955045345834197, 6.955235391828881, 6.955235391828882], [1.717256586073414, 3.417902492165059, 3.418289197696307, 4.006235499104553, 4.006565420335059, 4.518897199069926, 4.978519230751274, 4.9785192307512744, 5.789993797990992, 6.500547318827066, 6.500547318827066, 7.14092755186499], [0.5724702671600166, 4.218594591447799, 4.218907906097472, 4.218907906097472, 4.707908851637848, 4.707908851637848, 4.708189604133328, 4.708189604133328, 6.29570230146562, 6.29570230146562, 7.556939141082784, 7.556939141082784], [2.3599069305349962, 2.359906930534998, 3.7818313003520823, 3.78218079650641, 4.321198561255806, 5.235059146689257, 5.235059146689258, 6.011786350662305, 6.011786350662306, 6.012006214164183, 6.699052618294945, 6.699052618294945], [1.716948672837036, 3.41813452073373, 3.41813452073373, 4.518487674583966, 4.978678528168267, 4.978678528168268, 5.78967418343894, 5.78967418343894, 6.500465983839474, 6.500465983839474, 7.140853510871712, 7.140853510871712], [2.538149934071421, 2.5381499340714213, 3.287867168266403, 4.4207643886210155, 5.713965143212813, 5.713965143212813, 6.083964126541941, 6.083964126541942, 6.432921958285101, 6.432921958285102, 6.763900527781585, 6.763900527781585], [0.5724702671600171, 4.218907906097472, 4.218907906097472, 4.708189604133328, 4.708189604133328, 4.708470339888347, 4.708470339888347, 5.151205177121809, 5.151205177121809, 5.151461770211021, 6.2961221918699914, 6.955349416933167], [2.359682877746807, 3.152137165776393, 3.152556471343213, 3.7820410019202884, 3.7823904786980087, 4.799954686961216, 5.235463114028927, 5.636958031913642, 6.364827311893895, 6.699171003830835, 6.6993683084084115, 7.3223812102608905], [1.9547268638345623, 2.8620737470709985, 3.543541726701021, 4.113946207379071, 4.114267491346154, 4.614370902468288, 4.614657345750079, 5.065859043343244, 5.479794675188184, 5.8648116006021995, 6.226064610883469, 7.202091391883804], [1.0962773422257552, 3.7819012021667815, 3.7819012021667815, 4.320953845077256, 4.3212597381350575, 4.321259738135058, 4.800119910248539, 5.235362125116259, 5.636864236106813, 6.364744242542257, 7.322128485487463, 7.614553892797944], [2.5383582341904414, 2.538358234190442, 3.2876259459191286, 3.8960227645327192, 4.420883985919037, 4.420883985919038, 4.421182965009993, 5.713826345100761, 5.713826345100761, 6.433209615097384, 6.763978695041821, 6.763978695041821], [2.5381499340714204, 2.538149934071421, 3.287867168266403, 4.4207643886210155, 4.89016020199505, 5.713965143212812, 6.083964126541941, 6.083964126541941, 6.432921958285101, 6.432921958285101, 6.763900527781585, 6.763900527781585], [1.9548621002066449, 2.8617042578089213, 3.5439893172296992, 4.114010466179742, 4.114010466179743, 4.614714632272832, 5.065911227573018, 5.480084122893346, 5.864856675928745, 5.8648566759287455, 6.567516630040667, 6.567717889723939], [2.704671783205202, 2.704671783205202, 2.7051604477379065, 4.006367470857006, 4.518721693120581, 4.519014199249398, 4.519014199249399, 5.399742604022198, 6.1555103324767515, 6.15572506260369, 6.500628652797006, 7.1410015920905785], [2.3596828777468075, 3.152137165776393, 3.152556471343214, 3.7820410019202866, 3.7823904786980087, 4.32138208929536, 4.799954686961217, 5.235463114028928, 5.636958031913641, 6.364827311893896, 6.699171003830836, 6.699368308408412], [1.7172565860734132, 3.4179024921650596, 3.4182891976963083, 4.006235499104552, 4.518897199069926, 4.978519230751274, 4.9785192307512744, 5.789993797990992, 6.500547318827066, 6.500547318827067, 7.14092755186499, 7.141112650989596], [1.440623856787413, 3.2876259459191286, 3.896022764532719, 3.8960227645327192, 4.420883985919038, 4.420883985919038, 4.890268319676531, 5.713826345100761, 5.713826345100762, 6.763978695041821, 6.763978695041821, 7.079683383348169], [1.4404403417417921, 3.2879475717827327, 3.8956156214377975, 3.8959549103049618, 4.889943959460573, 5.317839538290181, 5.318088091423597, 5.713780078314155, 6.432963052902951, 6.763939611524621, 6.764135026852361, 7.07945933646696], [1.716948672837036, 3.4181345207337306, 3.4181345207337306, 4.0067633600336485, 4.0067633600336485, 4.978678528168267, 4.978678528168267, 4.978944012537487, 5.3997915615623775, 6.15555327910139, 6.15555327910139, 7.141223708161449], [2.360130962053329, 3.152053297969595, 3.152053297969595, 3.782320585925725, 3.782320585925726, 4.321015025421198, 4.799899611268254, 5.235412619816097, 6.364785777353597, 6.364993447344765, 6.699131542217993, 7.322164589560574], [1.9552677532010339, 2.861519495286735, 3.543467122782915, 4.113881947574675, 4.1142032365598995, 4.6146000585161575, 5.065545926675186, 5.479987642023664, 5.864766524929215, 6.567436124440425, 6.891957826114611, 7.499163761830804], [1.4404403417417924, 3.287947571782732, 3.895615621437797, 3.8959549103049618, 4.421123170809282, 4.889943959460572, 5.317839538290181, 5.713780078314154, 6.432963052902951, 6.76393961152462, 6.76413502685236, 7.07945933646696], [1.0962773422257543, 4.3212597381350575, 4.3212597381350575, 4.800119910248538, 4.80011991024854, 5.235362125116258, 5.235362125116259, 5.23561459374551, 5.637333199534894, 5.637333199534895, 7.017904766803825, 7.0179047668038255], [1.4404403417417908, 3.2879475717827322, 3.8959549103049627, 4.421123170809281, 4.421422133726416, 4.890484547868772, 5.318088091423597, 5.714011408500935, 5.714242729322756, 6.084224831875973, 7.079832743996675, 7.672011635786421], [1.0960361729658996, 3.78218079650641, 3.78218079650641, 4.321504436991634, 4.800064836451338, 4.800064836451339, 5.23556410099362, 5.23556410099362, 5.6370518261597855, 5.6370518261597855, 6.365118046087225, 7.614866345115637], [1.4404403417417915, 3.287947571782733, 3.895954910304962, 4.421123170809281, 4.421422133726417, 4.890484547868773, 5.318088091423596, 5.7140114085009355, 5.7142427293227565, 5.714242729322758, 6.084224831875973, 7.0798327439966755], [1.9548621002066449, 2.861704257808921, 3.543989317229698, 4.114010466179742, 4.114010466179743, 4.614714632272832, 5.480084122893346, 5.8648566759287455, 5.8648566759287455, 6.567516630040667, 6.567717889723938, 7.785009954544012], [1.716948672837034, 3.4181345207337306, 3.4181345207337315, 3.4185212000177447, 4.978678528168266, 4.978678528168267, 4.978944012537486, 4.978944012537486, 5.790130770255336, 6.1555532791013885, 6.1555532791013885, 7.7287002080997995], [3.0103813091037743, 3.0103813091037743, 3.010381309103776, 3.6650927202020234, 3.6650927202020243, 5.558931800974737, 5.558931800974738, 5.939043002821646, 7.2623033473943455, 7.2623033473943455, 7.5572189945145585, 7.557218994514559], [2.3596828777468075, 3.152137165776393, 3.152556471343213, 3.7820410019202875, 3.7823904786980087, 4.32138208929536, 4.799954686961217, 5.235463114028928, 5.636958031913641, 6.364827311893896, 6.699171003830836, 7.3223812102608905], [1.9552677532010343, 2.861519495286735, 3.5434671227829146, 4.113881947574676, 4.1142032365598995, 4.6146000585161575, 5.065545926675185, 5.479987642023664, 5.864991899829825, 6.567436124440425, 7.201871153060141, 7.784772248560299], [3.0102934919328925, 3.010732552172754, 3.010732552172755, 3.6646599209082007, 3.6646599209082016, 3.6650205905356184, 5.15130781589124, 5.558884244995609, 5.55888424499561, 6.955045345834196, 6.955045345834197, 6.955235391828882], [1.9552677532010332, 2.8615194952867355, 3.543467122782915, 4.113881947574675, 4.1142032365598995, 4.6146000585161575, 4.614600058516158, 5.065545926675186, 5.864766524929216, 6.567436124440425, 6.891957826114612, 7.499163761830804], [2.3601309620533297, 3.1520532979695948, 3.1520532979695948, 3.782320585925725, 4.321015025421197, 4.799899611268254, 5.235412619816098, 6.364785777353597, 6.364993447344765, 6.699131542217993, 7.322164589560574, 7.614762195767592], [1.096277342225755, 3.781901202166782, 3.781901202166782, 4.320953845077256, 4.80011991024854, 4.80011991024854, 5.235362125116258, 5.235362125116258, 6.364744242542257, 6.364744242542257, 8.16805740938438, 8.16805740938438], [1.7172565860734126, 3.4179024921650596, 3.4182891976963083, 4.006235499104552, 4.006565420335059, 4.518897199069926, 4.978519230751273, 4.9785192307512744, 6.500547318827066, 6.500547318827067, 7.14092755186499, 7.141112650989596], [1.0960361729658998, 3.7821807965064096, 3.782180796506411, 4.32089266386705, 4.320892663867051, 4.800064836451338, 5.235059146689257, 5.636817337618119, 5.6370518261597855, 7.0174903926561765, 7.322092381236329, 7.896123586674277], [1.9549973272237893, 2.8617966345967947, 3.5436909298254156, 4.113753424954532, 4.614199027963847, 4.614485481914714, 5.065441550151368, 5.864676372543897, 6.226149530500466, 6.567355617853308, 7.201797738622222, 7.498916994897432], [1.095794950628038, 3.782110899859236, 4.321137383510435, 4.321137383510436, 4.799734380397486, 5.235008648579964, 5.235261134255498, 5.636770438739225, 6.364661172106427, 7.0174527210658075, 7.614484457208423, 7.896090106971046], [1.9548621002066449, 2.8617042578089205, 4.114010466179741, 4.114010466179743, 4.614141735039648, 5.479601701557281, 5.864631295831548, 5.8648566759287455, 6.225894768174628, 6.891842752200527, 7.2017610311226194, 7.498881741815489], [1.7169486728370353, 3.4181345207337306, 3.4181345207337306, 4.518487674583966, 4.978678528168267, 5.789674183438939, 5.789674183438939, 6.500465983839474, 6.500465983839474, 6.500669319400369, 7.140853510871712, 7.140853510871712], [3.0103813091037743, 3.0103813091037743, 3.0103813091037748, 5.150845925322531, 5.5589318009747375, 5.5589318009747375, 6.9548933052994135, 6.9548933052994135, 6.9548933052994135, 6.9548933052994135, 6.9548933052994135, 6.9548933052994135], [1.096277342225754, 4.3212597381350575, 4.3212597381350575, 4.800119910248538, 4.80011991024854, 5.235362125116258, 5.235362125116259, 5.23561459374551, 5.637333199534894, 5.637333199534895, 7.017904766803825, 7.614901061248439], [1.4404403417417913, 3.287947571782733, 3.895954910304962, 4.421123170809281, 4.421422133726417, 4.890484547868773, 5.318088091423596, 5.714011408500935, 5.7142427293227565, 5.714242729322758, 6.084224831875973, 7.672011635786422], [2.53814993407142, 2.538149934071421, 3.2878671682664042, 3.8962263201257503, 4.421362342760207, 4.890160201995049, 5.713965143212813, 6.084398629226024, 6.7640959442384565, 7.07960870184225, 7.381826900752755, 7.951546972089884], [1.9548621002066446, 2.8617042578089213, 3.5439893172296983, 4.114010466179742, 4.114010466179742, 4.614714632272832, 5.065911227573018, 5.480084122893346, 5.8648566759287455, 5.8648566759287455, 6.567516630040667, 7.785009954544012], [2.7046717832052005, 2.7046717832052014, 2.7051604477379074, 4.006367470857006, 4.518721693120581, 4.519014199249398, 5.399742604022198, 6.155510332476751, 6.15572506260369, 6.500628652797005, 7.141001592090578, 8.006256529514367], [2.5380457776011314, 2.5385665172175553, 3.2877867627837887, 3.287786762783789, 4.890376434967719, 4.8903764349677195, 5.317988671564261, 5.317988671564262, 5.318237217727784, 6.764056861398736, 6.764056861398736, 7.951513725745808], [1.7172565860734137, 3.417902492165059, 3.418289197696309, 4.006235499104552, 4.0065654203350585, 4.978519230751274, 4.978519230751274, 5.399644687610174, 6.155639171451777, 7.140927551864989, 7.14092755186499, 8.006025392540087], [2.3600189489525167, 3.1523887558092056, 3.1523887558092074, 3.7819012021667815, 3.7819012021667824, 4.3209538450772556, 5.235362125116258, 5.636864236106814, 6.364744242542256, 6.6992893872746935, 7.322128485487464, 7.614553892797943], [0.5724702671600161, 4.218594591447799, 4.218907906097474, 4.707908851637847, 4.707908851637847, 4.708189604133327, 5.151205177121808, 5.151205177121808, 6.29570230146562, 6.954969325982269, 8.114373668910236, 8.379195991683279], [1.9549973272237886, 2.861796634596795, 3.543690929825416, 4.113753424954532, 4.614199027963848, 4.614485481914714, 5.06544155015137, 5.864676372543897, 6.567355617853309, 6.892072898107356, 7.201797738622222, 7.498916994897432], [1.9548621002066442, 2.861704257808921, 4.114010466179742, 4.114010466179743, 4.614141735039648, 5.47960170155728, 5.864631295831548, 6.225894768174627, 6.567516630040667, 6.891842752200528, 7.2017610311226194, 7.498881741815489], [2.3596828777468066, 3.152137165776393, 3.7820410019202866, 4.799954686961218, 5.23495814998355, 5.636958031913641, 6.364619636481925, 6.698973693442055, 6.698973693442055, 7.322020172199982, 7.322020172199982, 7.614449739176221], [2.360130962053329, 3.1520532979695948, 3.1520532979695948, 3.782320585925725, 3.782320585925726, 4.321015025421198, 4.799899611268254, 5.235412619816097, 6.364785777353597, 6.699131542217993, 7.322164589560574, 7.614762195767592], [1.4406238567874128, 3.8960227645327183, 3.8960227645327183, 4.89026831967653, 4.89026831967653, 5.318386339850504, 5.318386339850504, 5.714057673414461, 5.714057673414461, 6.084485526039419, 6.433415076374333, 7.672046093335863], [2.5381499340714213, 2.5381499340714213, 3.287867168266403, 3.8962263201257517, 4.421362342760207, 4.421362342760208, 4.89016020199505, 5.713965143212812, 6.084398629226025, 6.764095944238457, 7.079608701842251, 7.381826900752756], [2.3596828777468075, 3.152137165776393, 3.152556471343214, 3.7820410019202866, 3.7823904786980096, 4.321382089295359, 4.799954686961217, 6.012138128405919, 6.364827311893895, 7.0176034062139205, 7.0177917580991505, 7.6146233277543], [2.3596828777468075, 3.152137165776393, 3.1525564713432126, 3.782041001920288, 4.321382089295359, 4.799954686961217, 6.012138128405919, 6.364827311893896, 7.0176034062139205, 7.01779175809915, 7.6146233277543, 8.16828396135895], [2.7046717832052014, 2.7046717832052014, 2.7051604477379065, 4.006367470857006, 4.518721693120581, 4.519014199249398, 4.519014199249399, 5.399742604022198, 6.1555103324767515, 6.500628652797006, 7.141001592090578, 8.006256529514367], [1.4406238567874128, 3.287625945919129, 3.8960227645327197, 4.420883985919038, 4.420883985919038, 4.89026831967653, 5.713826345100761, 5.71405767341446, 5.714057673414461, 7.0794966781062225, 7.951280997444949, 8.482841526104558], [2.3600189489525167, 3.1523887558092065, 3.1523887558092074, 3.781901202166781, 3.781901202166781, 4.3209538450772556, 5.235362125116258, 5.636864236106813, 6.3647442425422565, 7.322128485487464, 7.322309004072833, 7.614553892797943], [1.0962773422257548, 3.781901202166782, 3.781901202166782, 4.320953845077256, 4.321259738135058, 4.800119910248539, 5.235362125116258, 5.636864236106814, 6.364744242542257, 7.322128485487464, 7.614553892797944, 7.896324461912696], [0.5724702671600164, 4.218594591447799, 4.218907906097473, 4.218907906097473, 4.707908851637847, 4.707908851637847, 4.708189604133328, 6.29570230146562, 6.29570230146562, 7.556939141082784, 7.556939141082784, 7.557114050692113], [2.359682877746807, 3.152137165776393, 3.7820410019202866, 4.799954686961218, 5.23495814998355, 6.364619636481925, 6.364827311893895, 6.698973693442055, 6.698973693442056, 7.322020172199982, 7.322020172199982, 7.614449739176221], [3.0103813091037748, 3.0103813091037748, 3.0103813091037748, 3.6650927202020247, 3.6650927202020247, 3.6650927202020256, 5.5589318009747375, 5.5589318009747375, 5.939043002821646, 7.262303347394346, 7.262303347394346, 7.557218994514559], [1.096277342225755, 3.7819012021667815, 3.7819012021667815, 4.320953845077256, 4.3212597381350575, 4.321259738135058, 4.800119910248539, 5.636864236106813, 6.364744242542257, 7.322128485487463, 7.614553892797943, 7.896324461912696], [2.166930463840415, 3.010556935760726, 3.0105569357607265, 4.708470339888347, 4.708470339888347, 5.151205177121808, 5.151205177121808, 5.151461770211021, 6.2961221918699914, 6.633730209328386, 6.633730209328386, 7.840949036733033], [2.538149934071421, 2.5381499340714213, 3.287867168266403, 3.896226320125751, 4.421362342760207, 4.421362342760208, 4.89016020199505, 5.713965143212812, 6.084398629226025, 6.764095944238457, 7.079608701842251, 7.951546972089884], [1.7174105219895281, 3.417979836771415, 3.417979836771415, 3.417979836771416, 4.978837820488555, 4.978837820488555, 4.978837820488555, 5.789811163264552, 5.789811163264553, 7.440513453247007, 7.440513453247008, 8.274507860054335], [2.5379416168562865, 2.5384623778402244, 3.2881083729171134, 3.8957513405305852, 4.420943783354774, 4.421242758402028, 4.890052081923117, 6.084311731171561, 6.7642131914027255, 7.079534019548522, 7.3815762112357985, 8.221390615175414], [3.010293491932892, 3.010732552172755, 3.010732552172756, 3.6646599209082007, 3.6646599209082007, 3.6650205905356175, 5.5588842449956095, 5.938998490548464, 6.295786281786824, 7.262448952253395, 7.557009105412317, 7.840679310341805], [1.9552677532010334, 2.8615194952867355, 3.5434671227829146, 4.113881947574676, 4.6146000585161575, 5.065545926675186, 5.479987642023664, 5.864991899829825, 6.567436124440425, 7.201871153060142, 7.784772248560299, 8.327127560675917], [1.0960361729658996, 3.78218079650641, 3.782180796506411, 4.32089266386705, 4.32089266386705, 4.800064836451338, 5.235059146689256, 5.636817337618119, 7.0174903926561765, 7.322092381236329, 7.614692762077511, 7.896123586674277], [1.0957949506280387, 3.782110899859236, 4.321137383510435, 4.321137383510436, 4.799734380397486, 5.235008648579964, 5.636770438739225, 6.364661172106427, 7.0174527210658075, 7.322236797172735, 7.614484457208423, 7.896090106971046], [2.3596828777468075, 3.152137165776393, 3.152556471343213, 3.7820410019202875, 3.782390478698009, 4.321382089295359, 4.799954686961217, 6.012138128405919, 6.364827311893895, 7.0176034062139205, 7.6146233277543, 8.16828396135895], [3.010293491932892, 3.010732552172754, 3.010732552172756, 3.6646599209082007, 3.6646599209082016, 3.6650205905356175, 5.558884244995609, 5.938998490548463, 6.295786281786824, 7.557009105412317, 7.840679310341805, 7.840847890423662], [1.9552677532010327, 2.8615194952867355, 3.5434671227829146, 4.113881947574675, 4.1142032365598995, 4.6146000585161575, 5.065545926675186, 5.479987642023663, 6.567436124440424, 7.201871153060142, 7.784772248560299, 8.327127560675917], [1.7172565860734124, 3.4179024921650596, 3.418289197696309, 4.006235499104552, 4.0065654203350585, 4.978519230751273, 4.9785192307512744, 5.399644687610174, 7.140927551864989, 7.14092755186499, 8.006025392540087, 8.006190491059764], [2.538149934071421, 2.5381499340714213, 3.287867168266403, 3.896226320125752, 4.421362342760207, 4.421362342760207, 5.713965143212812, 5.713965143212812, 6.764291355049861, 7.6718048872397215, 7.6718048872397215, 8.2216156975189], [2.3596828777468075, 3.152137165776393, 3.152556471343215, 3.7820410019202866, 3.7823904786980087, 4.321382089295359, 5.636958031913641, 6.364827311893895, 6.6993683084084115, 7.8962240249322555, 7.896391419189938, 8.168122139161163], [2.537941616856286, 2.5384623778402244, 3.288108372917113, 3.895751340530585, 4.420943783354774, 4.421242758402028, 4.890052081923117, 6.084311731171561, 7.079534019548522, 7.3815762112357985, 8.221390615175414, 8.483028508072508], [1.0962773422257541, 3.781901202166782, 3.781901202166782, 4.320953845077256, 4.80011991024854, 5.235362125116258, 5.235362125116258, 6.364744242542257, 6.364744242542257, 8.16805740938438, 8.16805740938438, 8.68651462283999], [0.5724702671600156, 4.218594591447799, 4.218907906097474, 4.707908851637847, 4.707908851637847, 4.708189604133327, 5.151205177121808, 6.29570230146562, 6.954969325982269, 8.114373668910236, 8.379195991683279, 8.379353737620837], [2.3596828777468075, 3.1521371657763924, 3.1525564713432144, 3.7820410019202866, 3.7823904786980083, 4.321382089295359, 5.636958031913641, 6.364827311893895, 6.6993683084084115, 7.8962240249322555, 8.168122139161163, 8.431413185328498], [1.4406238567874123, 3.2876259459191286, 3.8960227645327192, 4.420883985919037, 4.420883985919038, 4.89026831967653, 5.713826345100761, 5.71405767341446, 7.0794966781062225, 7.951280997444949, 8.482841526104558, 8.736653213815941]]
  out "Array 2":T2(array[cluster])=[[{"norm"=5.220157487653798, "Atomic Positions (Cartesian)"=[0.0, 9.913474271797499, 16.522457119662498]}, {"norm"=5.220157487653799, "Atomic Positions (Cartesian)"=[3.3044914239325, 6.608982847865, 16.522457119662498]}, {"norm"=5.2201574876537995, "Atomic Positions (Cartesian)"=[3.3044914239325, 9.913474271797499, 13.21796569573]}, {"norm"=5.220623632620093, "Atomic Positions (Cartesian)"=[0.0, 3.3044914239325, 16.522457119662498]}, {"norm"=5.220623632620094, "Atomic Positions (Cartesian)"=[-3.3044914239325003, 6.608982847865, 16.522457119662498]}, {"norm"=5.220623632620095, "Atomic Positions (Cartesian)"=[3.3044914239325, 3.3044914239325, 13.21796569573]}, {"norm"=5.220623632620096, "Atomic Positions (Cartesian)"=[-3.3044914239325003, 9.913474271797499, 13.21796569573]}, {"norm"=5.220623632620096, "Atomic Positions (Cartesian)"=[0.0, 9.913474271797499, 9.913474271797499]}, {"norm"=5.220623632620096, "Atomic Positions (Cartesian)"=[3.3044914239325, 6.608982847865, 9.913474271797499]}, {"norm"=5.221451153767244, "Atomic Positions (Cartesian)"=[-3.3044914239325003, 3.3044914239325, 13.21796569573]}, {"norm"=5.221451153767244, "Atomic Positions (Cartesian)"=[0.0, 3.3044914239325, 9.913474271797499]}, {"norm"=5.221451153767246, "Atomic Positions (Cartesian)"=[-3.3044914239325003, 6.608982847865, 9.913474271797499]}, {"norm"=7.025101807449438, "Atomic Positions (Cartesian)"=[0.0, 13.21796569573, 13.21796569573]}, {"norm"=7.025101807449438, "Atomic Positions (Cartesian)"=[6.608982847865, 6.608982847865, 13.21796569573]}, {"norm"=7.026048715813021, "Atomic Positions (Cartesian)"=[0.0, 0.0, 13.21796569573]}, {"norm"=7.026048715813022, "Atomic Positions (Cartesian)"=[0.0, 6.608982847865, 6.608982847865]}, {"norm"=8.44338246181125, "Atomic Positions (Cartesian)"=[-3.3044914239325003, 13.21796569573, 16.522457119662498]}, {"norm"=8.44338246181125, "Atomic Positions (Cartesian)"=[3.3044914239325, 13.21796569573, 9.913474271797499]}, {"norm"=8.44338246181125, "Atomic Positions (Cartesian)"=[6.608982847865, 3.3044914239325, 16.522457119662498]}, {"norm"=8.44338246181125, "Atomic Positions (Cartesian)"=[6.608982847865, 9.913474271797499, 9.913474271797499]}, {"norm"=8.443728052441013, "Atomic Positions (Cartesian)"=[3.3044914239325, 0.0, 16.522457119662498]}, {"norm"=8.443728052441015, "Atomic Positions (Cartesian)"=[3.3044914239325, 9.913474271797499, 6.608982847865]}, {"norm"=8.444607175794442, "Atomic Positions (Cartesian)"=[-3.3044914239325003, 0.0, 9.913474271797499]}, {"norm"=8.444607175794442, "Atomic Positions (Cartesian)"=[-3.3044914239325003, 3.3044914239325, 6.608982847865]}, {"norm"=9.141984792899562, "Atomic Positions (Cartesian)"=[6.608982847865, 3.3044914239325, 9.913474271797499]}, {"norm"=9.141984792899564, "Atomic Positions (Cartesian)"=[-3.3044914239325003, 13.21796569573, 9.913474271797499]}, {"norm"=9.142013703792253, "Atomic Positions (Cartesian)"=[3.3044914239325, 13.21796569573, 16.522457119662498]}, {"norm"=9.142013703792253, "Atomic Positions (Cartesian)"=[6.608982847865, 9.913474271797499, 16.522457119662498]}, {"norm"=9.143238479547174, "Atomic Positions (Cartesian)"=[-3.3044914239325003, 0.0, 16.522457119662498]}, {"norm"=9.143238479547174, "Atomic Positions (Cartesian)"=[-3.3044914239325003, 9.913474271797499, 6.608982847865]}, {"norm"=9.143238479547174, "Atomic Positions (Cartesian)"=[3.3044914239325, 0.0, 9.913474271797499]}, {"norm"=9.143238479547174, "Atomic Positions (Cartesian)"=[3.3044914239325, 3.3044914239325, 6.608982847865]}, {"norm"=9.893293515306882, "Atomic Positions (Cartesian)"=[6.608982847865, 13.21796569573, 13.21796569573]}, {"norm"=9.893880180969104, "Atomic Positions (Cartesian)"=[0.0, 13.21796569573, 6.608982847865]}, {"norm"=9.893880180969104, "Atomic Positions (Cartesian)"=[6.608982847865, 0.0, 13.21796569573]}, {"norm"=9.893880180969104, "Atomic Positions (Cartesian)"=[6.608982847865, 6.608982847865, 6.608982847865]}, {"norm"=9.894828276308065, "Atomic Positions (Cartesian)"=[0.0, 0.0, 6.608982847865]}, {"norm"=10.865652799459163, "Atomic Positions (Cartesian)"=[0.0, 16.522457119662498, 16.522457119662498]}, {"norm"=10.865652799459163, "Atomic Positions (Cartesian)"=[3.3044914239325, 16.522457119662498, 13.21796569573]}, {"norm"=10.865652799459163, "Atomic Positions (Cartesian)"=[9.913474271797499, 6.608982847865, 16.522457119662498]}, {"norm"=10.865652799459163, "Atomic Positions (Cartesian)"=[9.913474271797499, 9.913474271797499, 13.21796569573]}, {"norm"=10.866022133210251, "Atomic Positions (Cartesian)"=[-3.3044914239325003, 16.522457119662498, 13.21796569573]}, {"norm"=10.866022133210251, "Atomic Positions (Cartesian)"=[0.0, 16.522457119662498, 9.913474271797499]}, {"norm"=10.866022133210251, "Atomic Positions (Cartesian)"=[9.913474271797499, 3.3044914239325, 13.21796569573]}, {"norm"=10.866022133210251, "Atomic Positions (Cartesian)"=[9.913474271797499, 6.608982847865, 9.913474271797499]}, {"norm"=10.866601497109711, "Atomic Positions (Cartesian)"=[0.0, -3.3044914239325003, 16.522457119662498]}, {"norm"=10.866601497109713, "Atomic Positions (Cartesian)"=[0.0, 9.913474271797499, 3.3044914239325]}, {"norm"=10.866601497109713, "Atomic Positions (Cartesian)"=[3.3044914239325, -3.3044914239325003, 13.21796569573]}, {"norm"=10.866601497109713, "Atomic Positions (Cartesian)"=[3.3044914239325, 6.608982847865, 3.3044914239325]}, {"norm"=10.866970802151895, "Atomic Positions (Cartesian)"=[-3.3044914239325003, -3.3044914239325003, 13.21796569573]}, {"norm"=10.866970802151895, "Atomic Positions (Cartesian)"=[-3.3044914239325003, 6.608982847865, 3.3044914239325]}, {"norm"=10.866970802151895, "Atomic Positions (Cartesian)"=[0.0, -3.3044914239325003, 9.913474271797499]}, {"norm"=10.866970802151895, "Atomic Positions (Cartesian)"=[0.0, 3.3044914239325, 3.3044914239325]}, {"norm"=11.796278258867796, "Atomic Positions (Cartesian)"=[6.608982847865, 13.21796569573, 6.608982847865]}, {"norm"=12.495895130294148, "Atomic Positions (Cartesian)"=[6.608982847865, 0.0, 6.608982847865]}, {"norm"=12.671233650206785, "Atomic Positions (Cartesian)"=[6.608982847865, -3.3044914239325003, 16.522457119662498]}, {"norm"=12.672035407935685, "Atomic Positions (Cartesian)"=[-3.3044914239325003, 0.0, 3.3044914239325]}, {"norm"=12.672035407935686, "Atomic Positions (Cartesian)"=[-3.3044914239325003, -3.3044914239325003, 6.608982847865]}, {"norm"=12.910839930400824, "Atomic Positions (Cartesian)"=[6.608982847865, 16.522457119662498, 16.522457119662498]}, {"norm"=12.910839930400824, "Atomic Positions (Cartesian)"=[9.913474271797499, 13.21796569573, 16.522457119662498]}, {"norm"=12.911227673951695, "Atomic Positions (Cartesian)"=[6.608982847865, 16.522457119662498, 9.913474271797499]}, {"norm"=12.911227673951695, "Atomic Positions (Cartesian)"=[9.913474271797499, 13.21796569573, 9.913474271797499]}, {"norm"=12.911615491299742, "Atomic Positions (Cartesian)"=[3.3044914239325, 16.522457119662498, 6.608982847865]}, {"norm"=12.911615491299742, "Atomic Positions (Cartesian)"=[9.913474271797499, 0.0, 16.522457119662498]}, {"norm"=12.911615491299742, "Atomic Positions (Cartesian)"=[9.913474271797499, 9.913474271797499, 6.608982847865]}, {"norm"=12.911641740122839, "Atomic Positions (Cartesian)"=[-3.3044914239325003, 16.522457119662498, 6.608982847865]}, {"norm"=12.911641740122839, "Atomic Positions (Cartesian)"=[3.3044914239325, 13.21796569573, 3.3044914239325]}, {"norm"=12.911641740122839, "Atomic Positions (Cartesian)"=[6.608982847865, 9.913474271797499, 3.3044914239325]}, {"norm"=12.911641740122839, "Atomic Positions (Cartesian)"=[9.913474271797499, 0.0, 9.913474271797499]}, {"norm"=12.911641740122839, "Atomic Positions (Cartesian)"=[9.913474271797499, 3.3044914239325, 6.608982847865]}, {"norm"=12.912029466341547, "Atomic Positions (Cartesian)"=[-3.3044914239325003, 13.21796569573, 3.3044914239325]}, {"norm"=12.912029466341547, "Atomic Positions (Cartesian)"=[6.608982847865, -3.3044914239325003, 9.913474271797499]}, {"norm"=12.912029466341547, "Atomic Positions (Cartesian)"=[6.608982847865, 3.3044914239325, 3.3044914239325]}, {"norm"=12.912417266358556, "Atomic Positions (Cartesian)"=[3.3044914239325, -3.3044914239325003, 6.608982847865]}, {"norm"=12.912417266358556, "Atomic Positions (Cartesian)"=[3.3044914239325, 0.0, 3.3044914239325]}, {"norm"=13.634031544767947, "Atomic Positions (Cartesian)"=[13.21796569573, 6.608982847865, 13.21796569573]}, {"norm"=13.63508463639721, "Atomic Positions (Cartesian)"=[0.0, 6.608982847865, 0.0]}, {"norm"=14.274754372970358, "Atomic Positions (Cartesian)"=[-3.3044914239325003, 3.3044914239325, 0.0]}, {"norm"=14.36847282562259, "Atomic Positions (Cartesian)"=[9.913474271797499, 16.522457119662498, 13.21796569573]}, {"norm"=14.368472825622591, "Atomic Positions (Cartesian)"=[13.21796569573, 9.913474271797499, 16.522457119662498]}, {"norm"=14.369006913948152, "Atomic Positions (Cartesian)"=[13.21796569573, 3.3044914239325, 9.913474271797499]}, {"norm"=14.369273964813878, "Atomic Positions (Cartesian)"=[0.0, 16.522457119662498, 3.3044914239325]}, {"norm"=14.369273964813878, "Atomic Positions (Cartesian)"=[9.913474271797499, -3.3044914239325003, 13.21796569573]}, {"norm"=14.369273964813878, "Atomic Positions (Cartesian)"=[9.913474271797499, 6.608982847865, 3.3044914239325]}, {"norm"=14.369714014784302, "Atomic Positions (Cartesian)"=[3.3044914239325, 3.3044914239325, 0.0]}, {"norm"=14.369714014784304, "Atomic Positions (Cartesian)"=[-3.3044914239325003, 9.913474271797499, 0.0]}, {"norm"=14.369981053762654, "Atomic Positions (Cartesian)"=[0.0, -3.3044914239325003, 3.3044914239325]}, {"norm"=15.067810726902614, "Atomic Positions (Cartesian)"=[13.21796569573, 3.3044914239325, 16.522457119662498]}, {"norm"=15.067810726902616, "Atomic Positions (Cartesian)"=[13.21796569573, 9.913474271797499, 9.913474271797499]}, {"norm"=15.068517839626741, "Atomic Positions (Cartesian)"=[3.3044914239325, 9.913474271797499, 0.0]}, {"norm"=15.085764614488502, "Atomic Positions (Cartesian)"=[0.0, 0.0, 0.0]}, {"norm"=15.324831063618976, "Atomic Positions (Cartesian)"=[13.21796569573, 13.21796569573, 13.21796569573]}, {"norm"=15.32551930605461, "Atomic Positions (Cartesian)"=[13.21796569573, 0.0, 13.21796569573]}, {"norm"=15.32551930605461, "Atomic Positions (Cartesian)"=[13.21796569573, 6.608982847865, 6.608982847865]}, {"norm"=15.32584597220856, "Atomic Positions (Cartesian)"=[0.0, 13.21796569573, 0.0]}, {"norm"=15.32584597220856, "Atomic Positions (Cartesian)"=[6.608982847865, 6.608982847865, 0.0]}, {"norm"=15.915578100034844, "Atomic Positions (Cartesian)"=[9.913474271797499, 16.522457119662498, 6.608982847865]}, {"norm"=15.915844396780688, "Atomic Positions (Cartesian)"=[6.608982847865, 16.522457119662498, 3.3044914239325]}, {"norm"=15.915844396780688, "Atomic Positions (Cartesian)"=[9.913474271797499, 13.21796569573, 3.3044914239325]}, {"norm"=15.916217706582081, "Atomic Positions (Cartesian)"=[9.913474271797499, 0.0, 3.3044914239325]}, {"norm"=15.916217706582083, "Atomic Positions (Cartesian)"=[9.913474271797499, -3.3044914239325003, 6.608982847865]}, {"norm"=15.916483994529953, "Atomic Positions (Cartesian)"=[6.608982847865, -3.3044914239325003, 3.3044914239325]}, {"norm"=16.53804587731425, "Atomic Positions (Cartesian)"=[13.21796569573, 0.0, 6.608982847865]}, {"norm"=16.53851678841079, "Atomic Positions (Cartesian)"=[6.608982847865, 0.0, 0.0]}, {"norm"=17.086867630974155, "Atomic Positions (Cartesian)"=[-3.3044914239325003, -3.3044914239325003, 0.0]}, {"norm"=17.15575574609642, "Atomic Positions (Cartesian)"=[13.21796569573, 16.522457119662498, 16.522457119662498]}, {"norm"=17.156625149376747, "Atomic Positions (Cartesian)"=[13.21796569573, 3.3044914239325, 3.3044914239325]}, {"norm"=17.15662514937675, "Atomic Positions (Cartesian)"=[13.21796569573, -3.3044914239325003, 9.913474271797499]}, {"norm"=17.156778795319642, "Atomic Positions (Cartesian)"=[-3.3044914239325003, 16.522457119662498, 0.0]}, {"norm"=17.156778795319642, "Atomic Positions (Cartesian)"=[9.913474271797499, 3.3044914239325, 0.0]}, {"norm"=17.157213487509914, "Atomic Positions (Cartesian)"=[0.0, 3.3044914239325, -3.3044914239325003]}, {"norm"=17.157213487509914, "Atomic Positions (Cartesian)"=[3.3044914239325, -3.3044914239325003, 0.0]}, {"norm"=17.157213487509917, "Atomic Positions (Cartesian)"=[-3.3044914239325003, 6.608982847865, -3.3044914239325003]}, {"norm"=17.236302617772804, "Atomic Positions (Cartesian)"=[6.608982847865, 13.21796569573, 0.0]}, {"norm"=17.236739812989402, "Atomic Positions (Cartesian)"=[13.21796569573, 13.21796569573, 6.608982847865]}, {"norm"=17.396444880615974, "Atomic Positions (Cartesian)"=[13.21796569573, 16.522457119662498, 9.913474271797499]}, {"norm"=17.396444880615974, "Atomic Positions (Cartesian)"=[16.522457119662498, 6.608982847865, 16.522457119662498]}, {"norm"=17.396444880615974, "Atomic Positions (Cartesian)"=[16.522457119662498, 9.913474271797499, 13.21796569573]}, {"norm"=17.396761470323575, "Atomic Positions (Cartesian)"=[16.522457119662498, 3.3044914239325, 13.21796569573]}, {"norm"=17.396761470323575, "Atomic Positions (Cartesian)"=[16.522457119662498, 6.608982847865, 9.913474271797499]}, {"norm"=17.397033239292803, "Atomic Positions (Cartesian)"=[3.3044914239325, 16.522457119662498, 0.0]}, {"norm"=17.397033239292803, "Atomic Positions (Cartesian)"=[9.913474271797499, 9.913474271797499, 0.0]}, {"norm"=17.397078137323323, "Atomic Positions (Cartesian)"=[13.21796569573, -3.3044914239325003, 16.522457119662498]}, {"norm"=17.397078137323327, "Atomic Positions (Cartesian)"=[13.21796569573, 9.913474271797499, 3.3044914239325]}, {"norm"=17.39766648230414, "Atomic Positions (Cartesian)"=[0.0, 9.913474271797499, -3.3044914239325003]}, {"norm"=17.39766648230414, "Atomic Positions (Cartesian)"=[3.3044914239325, 6.608982847865, -3.3044914239325003]}, {"norm"=18.30985743635997, "Atomic Positions (Cartesian)"=[-3.3044914239325003, 0.0, -3.3044914239325003]}, {"norm"=18.35427016655129, "Atomic Positions (Cartesian)"=[3.3044914239325, 0.0, -3.3044914239325003]}, {"norm"=18.44809348568159, "Atomic Positions (Cartesian)"=[16.522457119662498, 13.21796569573, 16.522457119662498]}, {"norm"=18.448735211343113, "Atomic Positions (Cartesian)"=[16.522457119662498, 0.0, 9.913474271797499]}, {"norm"=18.448735211343113, "Atomic Positions (Cartesian)"=[16.522457119662498, 3.3044914239325, 6.608982847865]}, {"norm"=18.44928293113756, "Atomic Positions (Cartesian)"=[-3.3044914239325003, 13.21796569573, -3.3044914239325003]}, {"norm"=18.44928293113756, "Atomic Positions (Cartesian)"=[6.608982847865, 3.3044914239325, -3.3044914239325003]}, {"norm"=18.999985247933935, "Atomic Positions (Cartesian)"=[13.21796569573, 6.608982847865, 0.0]}, {"norm"=19.14656412810929, "Atomic Positions (Cartesian)"=[16.522457119662498, 13.21796569573, 9.913474271797499]}, {"norm"=19.14759215555354, "Atomic Positions (Cartesian)"=[16.522457119662498, 0.0, 16.522457119662498]}, {"norm"=19.14759215555354, "Atomic Positions (Cartesian)"=[16.522457119662498, 9.913474271797499, 6.608982847865]}, {"norm"=19.148139880873018, "Atomic Positions (Cartesian)"=[3.3044914239325, 13.21796569573, -3.3044914239325003]}, {"norm"=19.148139880873018, "Atomic Positions (Cartesian)"=[6.608982847865, 9.913474271797499, -3.3044914239325003]}, {"norm"=19.49086693515782, "Atomic Positions (Cartesian)"=[0.0, -3.3044914239325003, -3.3044914239325003]}, {"norm"=19.545399206799946, "Atomic Positions (Cartesian)"=[13.21796569573, -3.3044914239325003, 3.3044914239325]}, {"norm"=19.545586294466027, "Atomic Positions (Cartesian)"=[9.913474271797499, -3.3044914239325003, 0.0]}, {"norm"=19.6841042505146, "Atomic Positions (Cartesian)"=[16.522457119662498, 16.522457119662498, 13.21796569573]}, {"norm"=19.68455337924197, "Atomic Positions (Cartesian)"=[13.21796569573, 16.522457119662498, 3.3044914239325]}, {"norm"=19.684618757718162, "Atomic Positions (Cartesian)"=[9.913474271797499, 16.522457119662498, 0.0]}, {"norm"=19.684777971747327, "Atomic Positions (Cartesian)"=[16.522457119662498, -3.3044914239325003, 13.21796569573]}, {"norm"=19.684777971747327, "Atomic Positions (Cartesian)"=[16.522457119662498, 6.608982847865, 3.3044914239325]}, {"norm"=19.685067877286585, "Atomic Positions (Cartesian)"=[0.0, 16.522457119662498, -3.3044914239325003]}, {"norm"=19.685067877286585, "Atomic Positions (Cartesian)"=[9.913474271797499, 6.608982847865, -3.3044914239325003]}, {"norm"=20.08136857773698, "Atomic Positions (Cartesian)"=[13.21796569573, 0.0, 0.0]}, {"norm"=20.176254721170384, "Atomic Positions (Cartesian)"=[13.21796569573, 13.21796569573, 0.0]}, {"norm"=20.606660431209697, "Atomic Positions (Cartesian)"=[16.522457119662498, -3.3044914239325003, 6.608982847865]}, {"norm"=20.606660431209697, "Atomic Positions (Cartesian)"=[16.522457119662498, 0.0, 3.3044914239325]}, {"norm"=20.606975169775268, "Atomic Positions (Cartesian)"=[9.913474271797499, 0.0, -3.3044914239325003]}, {"norm"=20.60714708965936, "Atomic Positions (Cartesian)"=[6.608982847865, -3.3044914239325003, -3.3044914239325003]}, {"norm"=20.917133518618414, "Atomic Positions (Cartesian)"=[16.522457119662498, 16.522457119662498, 6.608982847865]}, {"norm"=20.917416211135077, "Atomic Positions (Cartesian)"=[16.522457119662498, 13.21796569573, 3.3044914239325]}, {"norm"=20.917620188694936, "Atomic Positions (Cartesian)"=[6.608982847865, 16.522457119662498, -3.3044914239325003]}, {"norm"=20.91762018869494, "Atomic Positions (Cartesian)"=[9.913474271797499, 13.21796569573, -3.3044914239325003]}, {"norm"=21.669829567990604, "Atomic Positions (Cartesian)"=[16.522457119662498, 3.3044914239325, 0.0]}, {"norm"=21.669959728186008, "Atomic Positions (Cartesian)"=[13.21796569573, 3.3044914239325, -3.3044914239325003]}, {"norm"=21.764870598252752, "Atomic Positions (Cartesian)"=[16.522457119662498, 9.913474271797499, 0.0]}, {"norm"=21.76496223420431, "Atomic Positions (Cartesian)"=[13.21796569573, 9.913474271797499, -3.3044914239325003]}, {"norm"=23.565725958168642, "Atomic Positions (Cartesian)"=[16.522457119662498, -3.3044914239325003, 0.0]}, {"norm"=23.56587319181664, "Atomic Positions (Cartesian)"=[13.21796569573, -3.3044914239325003, -3.3044914239325003]}, {"norm"=23.602690164823485, "Atomic Positions (Cartesian)"=[16.522457119662498, 6.608982847865, -3.3044914239325003]}, {"norm"=23.672916518917816, "Atomic Positions (Cartesian)"=[16.522457119662498, 16.522457119662498, 0.0]}, {"norm"=23.673015490129632, "Atomic Positions (Cartesian)"=[13.21796569573, 16.522457119662498, -3.3044914239325003]}, {"norm"=24.465589924042533, "Atomic Positions (Cartesian)"=[16.522457119662498, 0.0, -3.3044914239325003]}, {"norm"=24.537082896113102, "Atomic Positions (Cartesian)"=[16.522457119662498, 13.21796569573, -3.3044914239325003]}], [{"norm"=4.504434862113091, "Atomic Positions (Cartesian)"=[-3.3044914239325003, 6.608982847865, 16.522457119662498]}, {"norm"=4.504434862113093, "Atomic Positions (Cartesian)"=[-3.3044914239325003, 9.913474271797499, 13.21796569573]}, {"norm"=4.977261842417363, "Atomic Positions (Cartesian)"=[3.3044914239325, 6.608982847865, 16.522457119662498]}, {"norm"=4.9772618424173665, "Atomic Positions (Cartesian)"=[3.3044914239325, 9.913474271797499, 13.21796569573]}, {"norm"=5.354225920553604, "Atomic Positions (Cartesian)"=[0.0, 3.3044914239325, 16.522457119662498]}, {"norm"=5.354225920553606, "Atomic Positions (Cartesian)"=[0.0, 9.913474271797499, 9.913474271797499]}, {"norm"=6.110517621597898, "Atomic Positions (Cartesian)"=[0.0, 13.21796569573, 13.21796569573]}, {"norm"=6.110959729766714, "Atomic Positions (Cartesian)"=[3.3044914239325, 3.3044914239325, 13.21796569573]}, {"norm"=6.110959729766715, "Atomic Positions (Cartesian)"=[3.3044914239325, 6.608982847865, 9.913474271797499]}, {"norm"=6.111202370476378, "Atomic Positions (Cartesian)"=[-3.3044914239325003, 3.3044914239325, 13.21796569573]}, {"norm"=6.11120237047638, "Atomic Positions (Cartesian)"=[-3.3044914239325003, 6.608982847865, 9.913474271797499]}, {"norm"=6.580966740315636, "Atomic Positions (Cartesian)"=[0.0, 3.3044914239325, 9.913474271797499]}, {"norm"=7.1726766901760515, "Atomic Positions (Cartesian)"=[-3.3044914239325003, 13.21796569573, 16.522457119662498]}, {"norm"=7.6454777784429915, "Atomic Positions (Cartesian)"=[3.3044914239325, 13.21796569573, 16.522457119662498]}, {"norm"=7.6460613784078655, "Atomic Positions (Cartesian)"=[6.608982847865, 6.608982847865, 13.21796569573]}, {"norm"=8.28279610657209, "Atomic Positions (Cartesian)"=[3.3044914239325, 13.21796569573, 9.913474271797499]}, {"norm"=8.282929427516647, "Atomic Positions (Cartesian)"=[-3.3044914239325003, 13.21796569573, 9.913474271797499]}, {"norm"=8.283262087749062, "Atomic Positions (Cartesian)"=[0.0, 0.0, 13.21796569573]}, {"norm"=8.283262087749062, "Atomic Positions (Cartesian)"=[0.0, 6.608982847865, 6.608982847865]}, {"norm"=8.84800010860365, "Atomic Positions (Cartesian)"=[6.608982847865, 3.3044914239325, 16.522457119662498]}, {"norm"=8.848000108603651, "Atomic Positions (Cartesian)"=[6.608982847865, 9.913474271797499, 9.913474271797499]}, {"norm"=9.05611358550678, "Atomic Positions (Cartesian)"=[3.3044914239325, 0.0, 16.522457119662498]}, {"norm"=9.056113585506782, "Atomic Positions (Cartesian)"=[3.3044914239325, 9.913474271797499, 6.608982847865]}, {"norm"=9.510740980925679, "Atomic Positions (Cartesian)"=[0.0, 16.522457119662498, 16.522457119662498]}, {"norm"=9.511290830870722, "Atomic Positions (Cartesian)"=[6.608982847865, 3.3044914239325, 9.913474271797499]}, {"norm"=9.528707950383739, "Atomic Positions (Cartesian)"=[6.608982847865, 13.21796569573, 13.21796569573]}, {"norm"=9.52921105098212, "Atomic Positions (Cartesian)"=[-3.3044914239325003, 0.0, 16.522457119662498]}, {"norm"=9.529211050982122, "Atomic Positions (Cartesian)"=[-3.3044914239325003, 9.913474271797499, 6.608982847865]}, {"norm"=9.969223020047787, "Atomic Positions (Cartesian)"=[3.3044914239325, 16.522457119662498, 13.21796569573]}, {"norm"=9.969505378222859, "Atomic Positions (Cartesian)"=[-3.3044914239325003, 16.522457119662498, 13.21796569573]}, {"norm"=9.969588350971645, "Atomic Positions (Cartesian)"=[0.0, 13.21796569573, 6.608982847865]}, {"norm"=9.969870667574613, "Atomic Positions (Cartesian)"=[3.3044914239325, 0.0, 9.913474271797499]}, {"norm"=9.969870667574614, "Atomic Positions (Cartesian)"=[3.3044914239325, 3.3044914239325, 6.608982847865]}, {"norm"=9.97015299355102, "Atomic Positions (Cartesian)"=[-3.3044914239325003, 0.0, 9.913474271797499]}, {"norm"=9.970152993551022, "Atomic Positions (Cartesian)"=[-3.3044914239325003, 3.3044914239325, 6.608982847865]}, {"norm"=10.201392167789699, "Atomic Positions (Cartesian)"=[0.0, 16.522457119662498, 9.913474271797499]}, {"norm"=10.597767903043867, "Atomic Positions (Cartesian)"=[6.608982847865, 0.0, 13.21796569573]}, {"norm"=10.597767903043868, "Atomic Positions (Cartesian)"=[6.608982847865, 6.608982847865, 6.608982847865]}, {"norm"=11.070438941182838, "Atomic Positions (Cartesian)"=[9.913474271797499, 6.608982847865, 16.522457119662498]}, {"norm"=11.07043894118284, "Atomic Positions (Cartesian)"=[9.913474271797499, 9.913474271797499, 13.21796569573]}, {"norm"=11.39835436902499, "Atomic Positions (Cartesian)"=[9.913474271797499, 3.3044914239325, 13.21796569573]}, {"norm"=11.398354369024991, "Atomic Positions (Cartesian)"=[9.913474271797499, 6.608982847865, 9.913474271797499]}, {"norm"=11.398910594951154, "Atomic Positions (Cartesian)"=[0.0, 0.0, 6.608982847865]}, {"norm"=11.837733139785053, "Atomic Positions (Cartesian)"=[6.608982847865, 16.522457119662498, 16.522457119662498]}, {"norm"=11.838517613455721, "Atomic Positions (Cartesian)"=[0.0, -3.3044914239325003, 16.522457119662498]}, {"norm"=11.838517613455725, "Atomic Positions (Cartesian)"=[0.0, 9.913474271797499, 3.3044914239325]}, {"norm"=11.935280927967659, "Atomic Positions (Cartesian)"=[6.608982847865, 13.21796569573, 6.608982847865]}, {"norm"=11.935615975739866, "Atomic Positions (Cartesian)"=[3.3044914239325, -3.3044914239325003, 13.21796569573]}, {"norm"=11.935615975739866, "Atomic Positions (Cartesian)"=[3.3044914239325, 6.608982847865, 3.3044914239325]}, {"norm"=12.291144876606106, "Atomic Positions (Cartesian)"=[6.608982847865, 16.522457119662498, 9.913474271797499]}, {"norm"=12.29188765408282, "Atomic Positions (Cartesian)"=[0.0, -3.3044914239325003, 9.913474271797499]}, {"norm"=12.291887654082823, "Atomic Positions (Cartesian)"=[0.0, 3.3044914239325, 3.3044914239325]}, {"norm"=12.407766177753645, "Atomic Positions (Cartesian)"=[9.913474271797499, 13.21796569573, 16.522457119662498]}, {"norm"=12.408978546847544, "Atomic Positions (Cartesian)"=[-3.3044914239325003, -3.3044914239325003, 13.21796569573]}, {"norm"=12.408978546847546, "Atomic Positions (Cartesian)"=[-3.3044914239325003, 6.608982847865, 3.3044914239325]}, {"norm"=12.660305621550934, "Atomic Positions (Cartesian)"=[9.913474271797499, 13.21796569573, 9.913474271797499]}, {"norm"=12.660536552429202, "Atomic Positions (Cartesian)"=[3.3044914239325, 16.522457119662498, 6.608982847865]}, {"norm"=12.660568100891163, "Atomic Positions (Cartesian)"=[-3.3044914239325003, 16.522457119662498, 6.608982847865]}, {"norm"=13.133444648974288, "Atomic Positions (Cartesian)"=[9.913474271797499, 0.0, 16.522457119662498]}, {"norm"=13.133444648974288, "Atomic Positions (Cartesian)"=[9.913474271797499, 9.913474271797499, 6.608982847865]}, {"norm"=13.133640596942856, "Atomic Positions (Cartesian)"=[3.3044914239325, 13.21796569573, 3.3044914239325]}, {"norm"=13.335787616448048, "Atomic Positions (Cartesian)"=[6.608982847865, -3.3044914239325003, 16.522457119662498]}, {"norm"=13.33578761644805, "Atomic Positions (Cartesian)"=[6.608982847865, 9.913474271797499, 3.3044914239325]}, {"norm"=13.606656840097367, "Atomic Positions (Cartesian)"=[6.608982847865, 0.0, 6.608982847865]}, {"norm"=13.606656840097369, "Atomic Positions (Cartesian)"=[-3.3044914239325003, 13.21796569573, 3.3044914239325]}, {"norm"=13.803123184717865, "Atomic Positions (Cartesian)"=[9.913474271797499, 16.522457119662498, 13.21796569573]}, {"norm"=13.803338551512816, "Atomic Positions (Cartesian)"=[13.21796569573, 6.608982847865, 13.21796569573]}, {"norm"=13.803569929375866, "Atomic Positions (Cartesian)"=[9.913474271797499, 0.0, 9.913474271797499]}, {"norm"=13.803569929375866, "Atomic Positions (Cartesian)"=[9.913474271797499, 3.3044914239325, 6.608982847865]}, {"norm"=14.18488149724124, "Atomic Positions (Cartesian)"=[13.21796569573, 9.913474271797499, 16.522457119662498]}, {"norm"=14.185530388092916, "Atomic Positions (Cartesian)"=[6.608982847865, -3.3044914239325003, 9.913474271797499]}, {"norm"=14.185530388092916, "Atomic Positions (Cartesian)"=[6.608982847865, 3.3044914239325, 3.3044914239325]}, {"norm"=14.228943309021655, "Atomic Positions (Cartesian)"=[-3.3044914239325003, -3.3044914239325003, 6.608982847865]}, {"norm"=14.228943309021655, "Atomic Positions (Cartesian)"=[-3.3044914239325003, 0.0, 3.3044914239325]}, {"norm"=14.533752883523292, "Atomic Positions (Cartesian)"=[13.21796569573, 3.3044914239325, 16.522457119662498]}, {"norm"=14.533752883523292, "Atomic Positions (Cartesian)"=[13.21796569573, 9.913474271797499, 9.913474271797499]}, {"norm"=14.534130003413024, "Atomic Positions (Cartesian)"=[0.0, 16.522457119662498, 3.3044914239325]}, {"norm"=14.701909751941269, "Atomic Positions (Cartesian)"=[3.3044914239325, -3.3044914239325003, 6.608982847865]}, {"norm"=14.701909751941269, "Atomic Positions (Cartesian)"=[3.3044914239325, 0.0, 3.3044914239325]}, {"norm"=14.855480554780419, "Atomic Positions (Cartesian)"=[13.21796569573, 13.21796569573, 13.21796569573]}, {"norm"=14.856297362291357, "Atomic Positions (Cartesian)"=[0.0, 6.608982847865, 0.0]}, {"norm"=14.96236169201476, "Atomic Positions (Cartesian)"=[13.21796569573, 3.3044914239325, 9.913474271797499]}, {"norm"=15.242890023899054, "Atomic Positions (Cartesian)"=[9.913474271797499, -3.3044914239325003, 13.21796569573]}, {"norm"=15.242890023899056, "Atomic Positions (Cartesian)"=[9.913474271797499, 6.608982847865, 3.3044914239325]}, {"norm"=15.242968763471708, "Atomic Positions (Cartesian)"=[3.3044914239325, 9.913474271797499, 0.0]}, {"norm"=15.716288894984004, "Atomic Positions (Cartesian)"=[-3.3044914239325003, 9.913474271797499, 0.0]}, {"norm"=15.836014372233292, "Atomic Positions (Cartesian)"=[9.913474271797499, 16.522457119662498, 6.608982847865]}, {"norm"=15.836207821675139, "Atomic Positions (Cartesian)"=[13.21796569573, 0.0, 13.21796569573]}, {"norm"=15.83620782167514, "Atomic Positions (Cartesian)"=[13.21796569573, 6.608982847865, 6.608982847865]}, {"norm"=15.83639530664301, "Atomic Positions (Cartesian)"=[0.0, 13.21796569573, 0.0]}, {"norm"=15.836588736967995, "Atomic Positions (Cartesian)"=[3.3044914239325, 3.3044914239325, 0.0]}, {"norm"=15.83678218103428, "Atomic Positions (Cartesian)"=[-3.3044914239325003, 3.3044914239325, 0.0]}, {"norm"=16.18275612495805, "Atomic Positions (Cartesian)"=[6.608982847865, 16.522457119662498, 3.3044914239325]}, {"norm"=16.183321803535353, "Atomic Positions (Cartesian)"=[0.0, -3.3044914239325003, 3.3044914239325]}, {"norm"=16.192173798791643, "Atomic Positions (Cartesian)"=[9.913474271797499, 13.21796569573, 3.3044914239325]}, {"norm"=16.192406156013735, "Atomic Positions (Cartesian)"=[6.608982847865, 6.608982847865, 0.0]}, {"norm"=16.46543914709017, "Atomic Positions (Cartesian)"=[13.21796569573, 16.522457119662498, 16.522457119662498]}, {"norm"=16.757358451904896, "Atomic Positions (Cartesian)"=[13.21796569573, 13.21796569573, 6.608982847865]}, {"norm"=16.758085588907534, "Atomic Positions (Cartesian)"=[0.0, 0.0, 0.0]}, {"norm"=16.834759353994116, "Atomic Positions (Cartesian)"=[13.21796569573, 16.522457119662498, 9.913474271797499]}, {"norm"=17.087441812779037, "Atomic Positions (Cartesian)"=[16.522457119662498, 6.608982847865, 16.522457119662498]}, {"norm"=17.087441812779037, "Atomic Positions (Cartesian)"=[16.522457119662498, 9.913474271797499, 13.21796569573]}, {"norm"=17.087906953764787, "Atomic Positions (Cartesian)"=[6.608982847865, 13.21796569573, 0.0]}, {"norm"=17.560882300412278, "Atomic Positions (Cartesian)"=[9.913474271797499, -3.3044914239325003, 6.608982847865]}, {"norm"=17.560882300412278, "Atomic Positions (Cartesian)"=[9.913474271797499, 0.0, 3.3044914239325]}, {"norm"=17.629233703568342, "Atomic Positions (Cartesian)"=[16.522457119662498, 3.3044914239325, 13.21796569573]}, {"norm"=17.629233703568342, "Atomic Positions (Cartesian)"=[16.522457119662498, 6.608982847865, 9.913474271797499]}, {"norm"=17.629391167356196, "Atomic Positions (Cartesian)"=[13.21796569573, 0.0, 6.608982847865]}, {"norm"=17.62956955750122, "Atomic Positions (Cartesian)"=[-3.3044914239325003, 16.522457119662498, 0.0]}, {"norm"=17.629590562170307, "Atomic Positions (Cartesian)"=[3.3044914239325, 16.522457119662498, 0.0]}, {"norm"=17.937254636672083, "Atomic Positions (Cartesian)"=[16.522457119662498, 13.21796569573, 16.522457119662498]}, {"norm"=17.937849277628377, "Atomic Positions (Cartesian)"=[9.913474271797499, 9.913474271797499, 0.0]}, {"norm"=17.951638104294773, "Atomic Positions (Cartesian)"=[13.21796569573, -3.3044914239325003, 16.522457119662498]}, {"norm"=17.951638104294773, "Atomic Positions (Cartesian)"=[13.21796569573, 9.913474271797499, 3.3044914239325]}, {"norm"=18.189180926563566, "Atomic Positions (Cartesian)"=[13.21796569573, -3.3044914239325003, 9.913474271797499]}, {"norm"=18.189180926563566, "Atomic Positions (Cartesian)"=[13.21796569573, 3.3044914239325, 3.3044914239325]}, {"norm"=18.189364223662043, "Atomic Positions (Cartesian)"=[0.0, 9.913474271797499, -3.3044914239325003]}, {"norm"=18.41120263286058, "Atomic Positions (Cartesian)"=[6.608982847865, 0.0, 0.0]}, {"norm"=18.45867167889952, "Atomic Positions (Cartesian)"=[16.522457119662498, 13.21796569573, 9.913474271797499]}, {"norm"=18.459162192603063, "Atomic Positions (Cartesian)"=[9.913474271797499, 3.3044914239325, 0.0]}, {"norm"=18.459334660093482, "Atomic Positions (Cartesian)"=[3.3044914239325, 6.608982847865, -3.3044914239325003]}, {"norm"=18.459507141832017, "Atomic Positions (Cartesian)"=[-3.3044914239325003, 6.608982847865, -3.3044914239325003]}, {"norm"=18.51621175370868, "Atomic Positions (Cartesian)"=[0.0, 3.3044914239325, -3.3044914239325003]}, {"norm"=18.7489790646271, "Atomic Positions (Cartesian)"=[-3.3044914239325003, -3.3044914239325003, 0.0]}, {"norm"=19.08087451244825, "Atomic Positions (Cartesian)"=[16.522457119662498, 16.522457119662498, 13.21796569573]}, {"norm"=19.221361734024548, "Atomic Positions (Cartesian)"=[16.522457119662498, 0.0, 16.522457119662498]}, {"norm"=19.22136173402455, "Atomic Positions (Cartesian)"=[16.522457119662498, 9.913474271797499, 6.608982847865]}, {"norm"=19.222220629939855, "Atomic Positions (Cartesian)"=[3.3044914239325, -3.3044914239325003, 0.0]}, {"norm"=19.251965781517363, "Atomic Positions (Cartesian)"=[16.522457119662498, 0.0, 9.913474271797499]}, {"norm"=19.251965781517363, "Atomic Positions (Cartesian)"=[16.522457119662498, 3.3044914239325, 6.608982847865]}, {"norm"=19.2521009717154, "Atomic Positions (Cartesian)"=[3.3044914239325, 13.21796569573, -3.3044914239325003]}, {"norm"=19.25226825556833, "Atomic Positions (Cartesian)"=[-3.3044914239325003, 13.21796569573, -3.3044914239325003]}, {"norm"=19.556173663620232, "Atomic Positions (Cartesian)"=[6.608982847865, 9.913474271797499, -3.3044914239325003]}, {"norm"=19.758973526759814, "Atomic Positions (Cartesian)"=[13.21796569573, 16.522457119662498, 3.3044914239325]}, {"norm"=19.759429368169727, "Atomic Positions (Cartesian)"=[6.608982847865, 3.3044914239325, -3.3044914239325003]}, {"norm"=19.84260884335743, "Atomic Positions (Cartesian)"=[-3.3044914239325003, 0.0, -3.3044914239325003]}, {"norm"=20.01272750547521, "Atomic Positions (Cartesian)"=[9.913474271797499, 16.522457119662498, 0.0]}, {"norm"=20.01289024344857, "Atomic Positions (Cartesian)"=[13.21796569573, 6.608982847865, 0.0]}, {"norm"=20.013178968112655, "Atomic Positions (Cartesian)"=[3.3044914239325, 0.0, -3.3044914239325003]}, {"norm"=20.053815501286348, "Atomic Positions (Cartesian)"=[0.0, 16.522457119662498, -3.3044914239325003]}, {"norm"=20.74416809609346, "Atomic Positions (Cartesian)"=[16.522457119662498, -3.3044914239325003, 13.21796569573]}, {"norm"=20.74416809609346, "Atomic Positions (Cartesian)"=[16.522457119662498, 6.608982847865, 3.3044914239325]}, {"norm"=20.744612432183104, "Atomic Positions (Cartesian)"=[16.522457119662498, 16.522457119662498, 6.608982847865]}, {"norm"=20.74492970284774, "Atomic Positions (Cartesian)"=[13.21796569573, 13.21796569573, 0.0]}, {"norm"=20.745047576375907, "Atomic Positions (Cartesian)"=[9.913474271797499, 6.608982847865, -3.3044914239325003]}, {"norm"=21.03501758753559, "Atomic Positions (Cartesian)"=[13.21796569573, -3.3044914239325003, 3.3044914239325]}, {"norm"=21.21107368532581, "Atomic Positions (Cartesian)"=[6.608982847865, 16.522457119662498, -3.3044914239325003]}, {"norm"=21.211497679431865, "Atomic Positions (Cartesian)"=[0.0, -3.3044914239325003, -3.3044914239325003]}, {"norm"=21.4515215977449, "Atomic Positions (Cartesian)"=[9.913474271797499, 13.21796569573, -3.3044914239325003]}, {"norm"=21.45167654105136, "Atomic Positions (Cartesian)"=[13.21796569573, 0.0, 0.0]}, {"norm"=21.462880521008653, "Atomic Positions (Cartesian)"=[16.522457119662498, 13.21796569573, 3.3044914239325]}, {"norm"=21.46330813825611, "Atomic Positions (Cartesian)"=[9.913474271797499, -3.3044914239325003, 0.0]}, {"norm"=21.684807117764812, "Atomic Positions (Cartesian)"=[16.522457119662498, -3.3044914239325003, 6.608982847865]}, {"norm"=21.684807117764812, "Atomic Positions (Cartesian)"=[16.522457119662498, 0.0, 3.3044914239325]}, {"norm"=22.135396480267275, "Atomic Positions (Cartesian)"=[9.913474271797499, 0.0, -3.3044914239325003]}, {"norm"=22.414195902633807, "Atomic Positions (Cartesian)"=[6.608982847865, -3.3044914239325003, -3.3044914239325003]}, {"norm"=22.567883557590037, "Atomic Positions (Cartesian)"=[13.21796569573, 9.913474271797499, -3.3044914239325003]}, {"norm"=22.79792367708377, "Atomic Positions (Cartesian)"=[16.522457119662498, 3.3044914239325, 0.0]}, {"norm"=22.815838964222234, "Atomic Positions (Cartesian)"=[13.21796569573, 3.3044914239325, -3.3044914239325003]}, {"norm"=22.830925376860986, "Atomic Positions (Cartesian)"=[16.522457119662498, 9.913474271797499, 0.0]}, {"norm"=24.0670863005095, "Atomic Positions (Cartesian)"=[16.522457119662498, 16.522457119662498, 0.0]}, {"norm"=24.076363953911024, "Atomic Positions (Cartesian)"=[13.21796569573, 16.522457119662498, -3.3044914239325003]}, {"norm"=24.67712113914527, "Atomic Positions (Cartesian)"=[16.522457119662498, 6.608982847865, -3.3044914239325003]}, {"norm"=24.864879689127136, "Atomic Positions (Cartesian)"=[16.522457119662498, -3.3044914239325003, 0.0]}, {"norm"=25.058400633219257, "Atomic Positions (Cartesian)"=[13.21796569573, -3.3044914239325003, -3.3044914239325003]}, {"norm"=25.271729896497547, "Atomic Positions (Cartesian)"=[16.522457119662498, 13.21796569573, -3.3044914239325003]}, {"norm"=25.682039043401197, "Atomic Positions (Cartesian)"=[16.522457119662498, 0.0, -3.3044914239325003]}, {"norm"=2316.707079699211, "Atomic Positions (Cartesian)"=[6.608982847865, 9.913474271797499, 16.522457119662498]}, {"norm"=2326.3229007096206, "Atomic Positions (Cartesian)"=[6.608982847865, -3.3044914239325003, 3.3044914239325]}, {"norm"=0.0, "Atomic Positions (Cartesian)"=[]}], [{"norm"=4.207159809223251, "Atomic Positions (Cartesian)"=[-3.3044914239325003, 9.913474271797499, 13.21796569573]}, {"norm"=5.0361678112018975, "Atomic Positions (Cartesian)"=[3.3044914239325, 6.608982847865, 16.522457119662498]}, {"norm"=5.036391447491676, "Atomic Positions (Cartesian)"=[0.0, 3.3044914239325, 16.522457119662498]}, {"norm"=5.674800812537473, "Atomic Positions (Cartesian)"=[3.3044914239325, 9.913474271797499, 13.21796569573]}, {"norm"=5.675293017996864, "Atomic Positions (Cartesian)"=[-3.3044914239325003, 3.3044914239325, 13.21796569573]}, {"norm"=5.997131649294962, "Atomic Positions (Cartesian)"=[0.0, 9.913474271797499, 9.913474271797499]}, {"norm"=5.997361851577354, "Atomic Positions (Cartesian)"=[-3.3044914239325003, 6.608982847865, 9.913474271797499]}, {"norm"=6.49432003317205, "Atomic Positions (Cartesian)"=[0.0, 13.21796569573, 13.21796569573]}, {"norm"=6.494612323446722, "Atomic Positions (Cartesian)"=[3.3044914239325, 3.3044914239325, 13.21796569573]}, {"norm"=6.836891216663987, "Atomic Positions (Cartesian)"=[-3.3044914239325003, 13.21796569573, 16.522457119662498]}, {"norm"=6.966521625415805, "Atomic Positions (Cartesian)"=[3.3044914239325, 6.608982847865, 9.913474271797499]}, {"norm"=6.966671675756571, "Atomic Positions (Cartesian)"=[0.0, 3.3044914239325, 9.913474271797499]}, {"norm"=7.8781518085073685, "Atomic Positions (Cartesian)"=[3.3044914239325, 13.21796569573, 16.522457119662498]}, {"norm"=8.355395583472063, "Atomic Positions (Cartesian)"=[6.608982847865, 6.608982847865, 13.21796569573]}, {"norm"=8.355561504091776, "Atomic Positions (Cartesian)"=[0.0, 0.0, 13.21796569573]}, {"norm"=8.433315141139456, "Atomic Positions (Cartesian)"=[-3.3044914239325003, 13.21796569573, 9.913474271797499]}, {"norm"=8.80513570400867, "Atomic Positions (Cartesian)"=[0.0, 6.608982847865, 6.608982847865]}, {"norm"=8.921776756100325, "Atomic Positions (Cartesian)"=[6.608982847865, 9.913474271797499, 16.522457119662498]}, {"norm"=8.921994053242832, "Atomic Positions (Cartesian)"=[-3.3044914239325003, 0.0, 16.522457119662498]}, {"norm"=9.175887025681533, "Atomic Positions (Cartesian)"=[6.608982847865, 3.3044914239325, 16.522457119662498]}, {"norm"=9.175887025681535, "Atomic Positions (Cartesian)"=[3.3044914239325, 13.21796569573, 9.913474271797499]}, {"norm"=9.175936199800937, "Atomic Positions (Cartesian)"=[3.3044914239325, 0.0, 16.522457119662498]}, {"norm"=9.556545555046487, "Atomic Positions (Cartesian)"=[-3.3044914239325003, 9.913474271797499, 6.608982847865]}, {"norm"=9.666882016716654, "Atomic Positions (Cartesian)"=[0.0, 16.522457119662498, 16.522457119662498]}, {"norm"=9.96748156324748, "Atomic Positions (Cartesian)"=[6.608982847865, 9.913474271797499, 9.913474271797499]}, {"norm"=9.96783910592073, "Atomic Positions (Cartesian)"=[-3.3044914239325003, 0.0, 9.913474271797499]}, {"norm"=9.986719630467109, "Atomic Positions (Cartesian)"=[-3.3044914239325003, 16.522457119662498, 13.21796569573]}, {"norm"=9.986912526630242, "Atomic Positions (Cartesian)"=[3.3044914239325, 9.913474271797499, 6.608982847865]}, {"norm"=9.987197709699988, "Atomic Positions (Cartesian)"=[-3.3044914239325003, 3.3044914239325, 6.608982847865]}, {"norm"=10.305992192574355, "Atomic Positions (Cartesian)"=[6.608982847865, 3.3044914239325, 9.913474271797499]}, {"norm"=10.306056084225348, "Atomic Positions (Cartesian)"=[3.3044914239325, 0.0, 9.913474271797499]}, {"norm"=10.467577406263311, "Atomic Positions (Cartesian)"=[3.3044914239325, 3.3044914239325, 6.608982847865]}, {"norm"=10.475340586168246, "Atomic Positions (Cartesian)"=[6.608982847865, 13.21796569573, 13.21796569573]}, {"norm"=10.629156575721709, "Atomic Positions (Cartesian)"=[3.3044914239325, 16.522457119662498, 13.21796569573]}, {"norm"=10.62937704973509, "Atomic Positions (Cartesian)"=[0.0, 13.21796569573, 6.608982847865]}, {"norm"=10.75381458396455, "Atomic Positions (Cartesian)"=[0.0, 16.522457119662498, 9.913474271797499]}, {"norm"=11.037907349344778, "Atomic Positions (Cartesian)"=[6.608982847865, 0.0, 13.21796569573]}, {"norm"=11.60660395421001, "Atomic Positions (Cartesian)"=[6.608982847865, 6.608982847865, 6.608982847865]}, {"norm"=11.6068224855672, "Atomic Positions (Cartesian)"=[0.0, 0.0, 6.608982847865]}, {"norm"=11.809623066876426, "Atomic Positions (Cartesian)"=[9.913474271797499, 6.608982847865, 16.522457119662498]}, {"norm"=11.809676367695047, "Atomic Positions (Cartesian)"=[0.0, -3.3044914239325003, 16.522457119662498]}, {"norm"=12.206953227456397, "Atomic Positions (Cartesian)"=[9.913474271797499, 3.3044914239325, 13.21796569573]}, {"norm"=12.207080824319737, "Atomic Positions (Cartesian)"=[3.3044914239325, -3.3044914239325003, 13.21796569573]}, {"norm"=12.550942544815165, "Atomic Positions (Cartesian)"=[6.608982847865, 16.522457119662498, 16.522457119662498]}, {"norm"=12.55139821586028, "Atomic Positions (Cartesian)"=[9.913474271797499, 6.608982847865, 9.913474271797499]}, {"norm"=12.551411500809957, "Atomic Positions (Cartesian)"=[0.0, 9.913474271797499, 3.3044914239325]}, {"norm"=12.551639279876335, "Atomic Positions (Cartesian)"=[-3.3044914239325003, 6.608982847865, 3.3044914239325]}, {"norm"=12.551639279876335, "Atomic Positions (Cartesian)"=[0.0, -3.3044914239325003, 9.913474271797499]}, {"norm"=12.770577419941814, "Atomic Positions (Cartesian)"=[3.3044914239325, 6.608982847865, 3.3044914239325]}, {"norm"=12.770737627626271, "Atomic Positions (Cartesian)"=[0.0, 3.3044914239325, 3.3044914239325]}, {"norm"=12.892155822527306, "Atomic Positions (Cartesian)"=[-3.3044914239325003, -3.3044914239325003, 13.21796569573]}, {"norm"=12.892973612825383, "Atomic Positions (Cartesian)"=[9.913474271797499, 9.913474271797499, 13.21796569573]}, {"norm"=13.040245318947033, "Atomic Positions (Cartesian)"=[-3.3044914239325003, 16.522457119662498, 6.608982847865]}, {"norm"=13.04025496195285, "Atomic Positions (Cartesian)"=[6.608982847865, 13.21796569573, 6.608982847865]}, {"norm"=13.327004417528801, "Atomic Positions (Cartesian)"=[6.608982847865, 16.522457119662498, 9.913474271797499]}, {"norm"=13.351138995646687, "Atomic Positions (Cartesian)"=[3.3044914239325, 16.522457119662498, 6.608982847865]}, {"norm"=13.589923423986582, "Atomic Positions (Cartesian)"=[9.913474271797499, 0.0, 16.522457119662498]}, {"norm"=13.589968457306272, "Atomic Positions (Cartesian)"=[6.608982847865, -3.3044914239325003, 16.522457119662498]}, {"norm"=13.833577360763394, "Atomic Positions (Cartesian)"=[6.608982847865, 0.0, 6.608982847865]}, {"norm"=14.055399806701555, "Atomic Positions (Cartesian)"=[9.913474271797499, 13.21796569573, 16.522457119662498]}, {"norm"=14.078566579409069, "Atomic Positions (Cartesian)"=[-3.3044914239325003, 13.21796569573, 3.3044914239325]}, {"norm"=14.078591664618525, "Atomic Positions (Cartesian)"=[9.913474271797499, 13.21796569573, 9.913474271797499]}, {"norm"=14.086053046355255, "Atomic Positions (Cartesian)"=[3.3044914239325, 13.21796569573, 3.3044914239325]}, {"norm"=14.356611524003767, "Atomic Positions (Cartesian)"=[9.913474271797499, 9.913474271797499, 6.608982847865]}, {"norm"=14.357039089549941, "Atomic Positions (Cartesian)"=[-3.3044914239325003, -3.3044914239325003, 6.608982847865]}, {"norm"=14.365054869577436, "Atomic Positions (Cartesian)"=[6.608982847865, 9.913474271797499, 3.3044914239325]}, {"norm"=14.365054869577438, "Atomic Positions (Cartesian)"=[9.913474271797499, 0.0, 9.913474271797499]}, {"norm"=14.365108461315602, "Atomic Positions (Cartesian)"=[6.608982847865, -3.3044914239325003, 9.913474271797499]}, {"norm"=14.365377312783625, "Atomic Positions (Cartesian)"=[-3.3044914239325003, 0.0, 3.3044914239325]}, {"norm"=14.588891282221704, "Atomic Positions (Cartesian)"=[9.913474271797499, 3.3044914239325, 6.608982847865]}, {"norm"=14.589064208061021, "Atomic Positions (Cartesian)"=[3.3044914239325, -3.3044914239325003, 6.608982847865]}, {"norm"=14.81808475457371, "Atomic Positions (Cartesian)"=[6.608982847865, 3.3044914239325, 3.3044914239325]}, {"norm"=14.8182258190618, "Atomic Positions (Cartesian)"=[3.3044914239325, 0.0, 3.3044914239325]}, {"norm"=15.077114117033357, "Atomic Positions (Cartesian)"=[9.913474271797499, 16.522457119662498, 13.21796569573]}, {"norm"=15.077431607633876, "Atomic Positions (Cartesian)"=[13.21796569573, 6.608982847865, 13.21796569573]}, {"norm"=15.314113181053907, "Atomic Positions (Cartesian)"=[13.21796569573, 3.3044914239325, 16.522457119662498]}, {"norm"=15.314180863442584, "Atomic Positions (Cartesian)"=[0.0, 16.522457119662498, 3.3044914239325]}, {"norm"=15.609910470685293, "Atomic Positions (Cartesian)"=[9.913474271797499, -3.3044914239325003, 13.21796569573]}, {"norm"=15.610517902308773, "Atomic Positions (Cartesian)"=[0.0, 6.608982847865, 0.0]}, {"norm"=15.966843684968655, "Atomic Positions (Cartesian)"=[13.21796569573, 3.3044914239325, 9.913474271797499]}, {"norm"=16.0103341060458, "Atomic Positions (Cartesian)"=[13.21796569573, 9.913474271797499, 9.913474271797499]}, {"norm"=16.102983719531174, "Atomic Positions (Cartesian)"=[13.21796569573, 9.913474271797499, 16.522457119662498]}, {"norm"=16.198707074849864, "Atomic Positions (Cartesian)"=[9.913474271797499, 6.608982847865, 3.3044914239325]}, {"norm"=16.198988357267787, "Atomic Positions (Cartesian)"=[0.0, -3.3044914239325003, 3.3044914239325]}, {"norm"=16.21343426829988, "Atomic Positions (Cartesian)"=[3.3044914239325, 9.913474271797499, 0.0]}, {"norm"=16.213750104195732, "Atomic Positions (Cartesian)"=[-3.3044914239325003, 3.3044914239325, 0.0]}, {"norm"=16.40016387784357, "Atomic Positions (Cartesian)"=[13.21796569573, 0.0, 13.21796569573]}, {"norm"=16.400433894152275, "Atomic Positions (Cartesian)"=[3.3044914239325, 3.3044914239325, 0.0]}, {"norm"=16.825987006525555, "Atomic Positions (Cartesian)"=[9.913474271797499, 16.522457119662498, 6.608982847865]}, {"norm"=16.82612367212332, "Atomic Positions (Cartesian)"=[13.21796569573, 6.608982847865, 6.608982847865]}, {"norm"=16.850754661141124, "Atomic Positions (Cartesian)"=[6.608982847865, 16.522457119662498, 3.3044914239325]}, {"norm"=16.888762886283384, "Atomic Positions (Cartesian)"=[0.0, 13.21796569573, 0.0]}, {"norm"=17.024208113946898, "Atomic Positions (Cartesian)"=[13.21796569573, 13.21796569573, 13.21796569573]}, {"norm"=17.02474885297415, "Atomic Positions (Cartesian)"=[-3.3044914239325003, 9.913474271797499, 0.0]}, {"norm"=17.039993811111536, "Atomic Positions (Cartesian)"=[6.608982847865, 6.608982847865, 0.0]}, {"norm"=17.040224656129347, "Atomic Positions (Cartesian)"=[0.0, 0.0, 0.0]}, {"norm"=17.232825491353374, "Atomic Positions (Cartesian)"=[9.913474271797499, 13.21796569573, 3.3044914239325]}, {"norm"=17.720922777259794, "Atomic Positions (Cartesian)"=[13.21796569573, 16.522457119662498, 16.522457119662498]}, {"norm"=17.87173186363254, "Atomic Positions (Cartesian)"=[13.21796569573, 13.21796569573, 6.608982847865]}, {"norm"=17.871914122574687, "Atomic Positions (Cartesian)"=[9.913474271797499, -3.3044914239325003, 6.608982847865]}, {"norm"=18.026156270619776, "Atomic Positions (Cartesian)"=[6.608982847865, 13.21796569573, 0.0]}, {"norm"=18.088951765336578, "Atomic Positions (Cartesian)"=[13.21796569573, -3.3044914239325003, 16.522457119662498]}, {"norm"=18.140622463899202, "Atomic Positions (Cartesian)"=[16.522457119662498, 6.608982847865, 16.522457119662498]}, {"norm"=18.140622463899206, "Atomic Positions (Cartesian)"=[13.21796569573, 16.522457119662498, 9.913474271797499]}, {"norm"=18.14091284109098, "Atomic Positions (Cartesian)"=[9.913474271797499, 0.0, 3.3044914239325]}, {"norm"=18.141095978265486, "Atomic Positions (Cartesian)"=[6.608982847865, -3.3044914239325003, 3.3044914239325]}, {"norm"=18.42130032908741, "Atomic Positions (Cartesian)"=[16.522457119662498, 3.3044914239325, 13.21796569573]}, {"norm"=18.421378707469557, "Atomic Positions (Cartesian)"=[3.3044914239325, 16.522457119662498, 0.0]}, {"norm"=18.42137870746956, "Atomic Positions (Cartesian)"=[13.21796569573, 0.0, 6.608982847865]}, {"norm"=18.514548020147803, "Atomic Positions (Cartesian)"=[16.522457119662498, 9.913474271797499, 13.21796569573]}, {"norm"=18.51472276673414, "Atomic Positions (Cartesian)"=[-3.3044914239325003, 16.522457119662498, 0.0]}, {"norm"=18.643966913730523, "Atomic Positions (Cartesian)"=[16.522457119662498, 6.608982847865, 9.913474271797499]}, {"norm"=18.785216383515973, "Atomic Positions (Cartesian)"=[13.21796569573, 9.913474271797499, 3.3044914239325]}, {"norm"=18.78522590974004, "Atomic Positions (Cartesian)"=[13.21796569573, -3.3044914239325003, 9.913474271797499]}, {"norm"=18.841792947117074, "Atomic Positions (Cartesian)"=[9.913474271797499, 9.913474271797499, 0.0]}, {"norm"=18.842140310151944, "Atomic Positions (Cartesian)"=[-3.3044914239325003, -3.3044914239325003, 0.0]}, {"norm"=18.90665143943113, "Atomic Positions (Cartesian)"=[6.608982847865, 0.0, 0.0]}, {"norm"=19.16794186392027, "Atomic Positions (Cartesian)"=[13.21796569573, 3.3044914239325, 3.3044914239325]}, {"norm"=19.168189730887242, "Atomic Positions (Cartesian)"=[3.3044914239325, 6.608982847865, -3.3044914239325003]}, {"norm"=19.168313674751005, "Atomic Positions (Cartesian)"=[0.0, 3.3044914239325, -3.3044914239325003]}, {"norm"=19.27333860147554, "Atomic Positions (Cartesian)"=[16.522457119662498, 13.21796569573, 16.522457119662498]}, {"norm"=19.274079222503445, "Atomic Positions (Cartesian)"=[0.0, 9.913474271797499, -3.3044914239325003]}, {"norm"=19.274370051615563, "Atomic Positions (Cartesian)"=[-3.3044914239325003, 6.608982847865, -3.3044914239325003]}, {"norm"=19.3407066609984, "Atomic Positions (Cartesian)"=[16.522457119662498, 0.0, 16.522457119662498]}, {"norm"=19.384670793597646, "Atomic Positions (Cartesian)"=[9.913474271797499, 3.3044914239325, 0.0]}, {"norm"=19.38495097420303, "Atomic Positions (Cartesian)"=[3.3044914239325, -3.3044914239325003, 0.0]}, {"norm"=19.64086385193392, "Atomic Positions (Cartesian)"=[16.522457119662498, 13.21796569573, 9.913474271797499]}, {"norm"=19.884360752506016, "Atomic Positions (Cartesian)"=[16.522457119662498, 0.0, 9.913474271797499]}, {"norm"=19.885694114278454, "Atomic Positions (Cartesian)"=[16.522457119662498, 9.913474271797499, 6.608982847865]}, {"norm"=20.048026939775532, "Atomic Positions (Cartesian)"=[16.522457119662498, 3.3044914239325, 6.608982847865]}, {"norm"=20.097123617281326, "Atomic Positions (Cartesian)"=[3.3044914239325, 13.21796569573, -3.3044914239325003]}, {"norm"=20.21632658974029, "Atomic Positions (Cartesian)"=[6.608982847865, 9.913474271797499, -3.3044914239325003]}, {"norm"=20.216637369898425, "Atomic Positions (Cartesian)"=[-3.3044914239325003, 0.0, -3.3044914239325003]}, {"norm"=20.347914530698134, "Atomic Positions (Cartesian)"=[16.522457119662498, 16.522457119662498, 13.21796569573]}, {"norm"=20.578149366126183, "Atomic Positions (Cartesian)"=[6.608982847865, 3.3044914239325, -3.3044914239325003]}, {"norm"=20.57826708742532, "Atomic Positions (Cartesian)"=[3.3044914239325, 0.0, -3.3044914239325003]}, {"norm"=20.730567486195984, "Atomic Positions (Cartesian)"=[13.21796569573, 16.522457119662498, 3.3044914239325]}, {"norm"=20.89424279741048, "Atomic Positions (Cartesian)"=[9.913474271797499, 16.522457119662498, 0.0]}, {"norm"=20.89424279741048, "Atomic Positions (Cartesian)"=[16.522457119662498, -3.3044914239325003, 13.21796569573]}, {"norm"=20.89424305278096, "Atomic Positions (Cartesian)"=[13.21796569573, 6.608982847865, 0.0]}, {"norm"=20.97988709707715, "Atomic Positions (Cartesian)"=[-3.3044914239325003, 13.21796569573, -3.3044914239325003]}, {"norm"=21.030967180431723, "Atomic Positions (Cartesian)"=[0.0, 16.522457119662498, -3.3044914239325003]}, {"norm"=21.236429139109894, "Atomic Positions (Cartesian)"=[16.522457119662498, 6.608982847865, 3.3044914239325]}, {"norm"=21.5506130018377, "Atomic Positions (Cartesian)"=[9.913474271797499, 6.608982847865, -3.3044914239325003]}, {"norm"=21.55090796591692, "Atomic Positions (Cartesian)"=[0.0, -3.3044914239325003, -3.3044914239325003]}, {"norm"=21.58773844899709, "Atomic Positions (Cartesian)"=[13.21796569573, 13.21796569573, 0.0]}, {"norm"=21.716881426166694, "Atomic Positions (Cartesian)"=[16.522457119662498, 16.522457119662498, 6.608982847865]}, {"norm"=22.031334935818418, "Atomic Positions (Cartesian)"=[16.522457119662498, 13.21796569573, 3.3044914239325]}, {"norm"=22.031519995908017, "Atomic Positions (Cartesian)"=[6.608982847865, 16.522457119662498, -3.3044914239325003]}, {"norm"=22.039065523437806, "Atomic Positions (Cartesian)"=[13.21796569573, -3.3044914239325003, 3.3044914239325]}, {"norm"=22.22057092919515, "Atomic Positions (Cartesian)"=[9.913474271797499, 13.21796569573, -3.3044914239325003]}, {"norm"=22.52418287971335, "Atomic Positions (Cartesian)"=[16.522457119662498, -3.3044914239325003, 6.608982847865]}, {"norm"=22.675554008096274, "Atomic Positions (Cartesian)"=[13.21796569573, 0.0, 0.0]}, {"norm"=22.718683803161536, "Atomic Positions (Cartesian)"=[16.522457119662498, 0.0, 3.3044914239325]}, {"norm"=23.002603424519243, "Atomic Positions (Cartesian)"=[9.913474271797499, -3.3044914239325003, 0.0]}, {"norm"=23.29422400396361, "Atomic Positions (Cartesian)"=[9.913474271797499, 0.0, -3.3044914239325003]}, {"norm"=23.294498670711768, "Atomic Positions (Cartesian)"=[6.608982847865, -3.3044914239325003, -3.3044914239325003]}, {"norm"=23.407176437297192, "Atomic Positions (Cartesian)"=[16.522457119662498, 9.913474271797499, 0.0]}, {"norm"=23.434128146099646, "Atomic Positions (Cartesian)"=[13.21796569573, 9.913474271797499, -3.3044914239325003]}, {"norm"=23.73124112534906, "Atomic Positions (Cartesian)"=[16.522457119662498, 3.3044914239325, 0.0]}, {"norm"=23.919469474392184, "Atomic Positions (Cartesian)"=[13.21796569573, 3.3044914239325, -3.3044914239325003]}, {"norm"=24.984038337947034, "Atomic Positions (Cartesian)"=[16.522457119662498, 16.522457119662498, 0.0]}, {"norm"=25.124670841391627, "Atomic Positions (Cartesian)"=[13.21796569573, 16.522457119662498, -3.3044914239325003]}, {"norm"=25.53316000735151, "Atomic Positions (Cartesian)"=[16.522457119662498, 6.608982847865, -3.3044914239325003]}, {"norm"=26.159742008541187, "Atomic Positions (Cartesian)"=[16.522457119662498, -3.3044914239325003, 0.0]}, {"norm"=26.206183663545936, "Atomic Positions (Cartesian)"=[16.522457119662498, 13.21796569573, -3.3044914239325003]}, {"norm"=26.896776750038075, "Atomic Positions (Cartesian)"=[16.522457119662498, 0.0, -3.3044914239325003]}, {"norm"=27.102340217486727, "Atomic Positions (Cartesian)"=[13.21796569573, -3.3044914239325003, -3.3044914239325003]}, {"norm"=0.0, "Atomic Positions (Cartesian)"=[]}, {"norm"=0.0, "Atomic Positions (Cartesian)"=[]}]]
  out "Array":dbl[][](array[numeric])=[[0.001, 6.609982847865, 13.218965695729999], [0.0, 6.608982847865, 13.21796569573], [0.0, 9.913474271797499, 16.522457119662498], [-3.3044914239325003, 6.608982847865, 16.522457119662498], [-3.3044914239325003, 9.913474271797499, 13.21796569573]]
  out "subarray":dbl[][](array[numeric])=[[0.0, 6.608982847865, 13.21796569573], [0.0, 9.913474271797499, 16.522457119662498], [-3.3044914239325003, 6.608982847865, 16.522457119662498], [-3.3044914239325003, 9.913474271797499, 13.21796569573]]
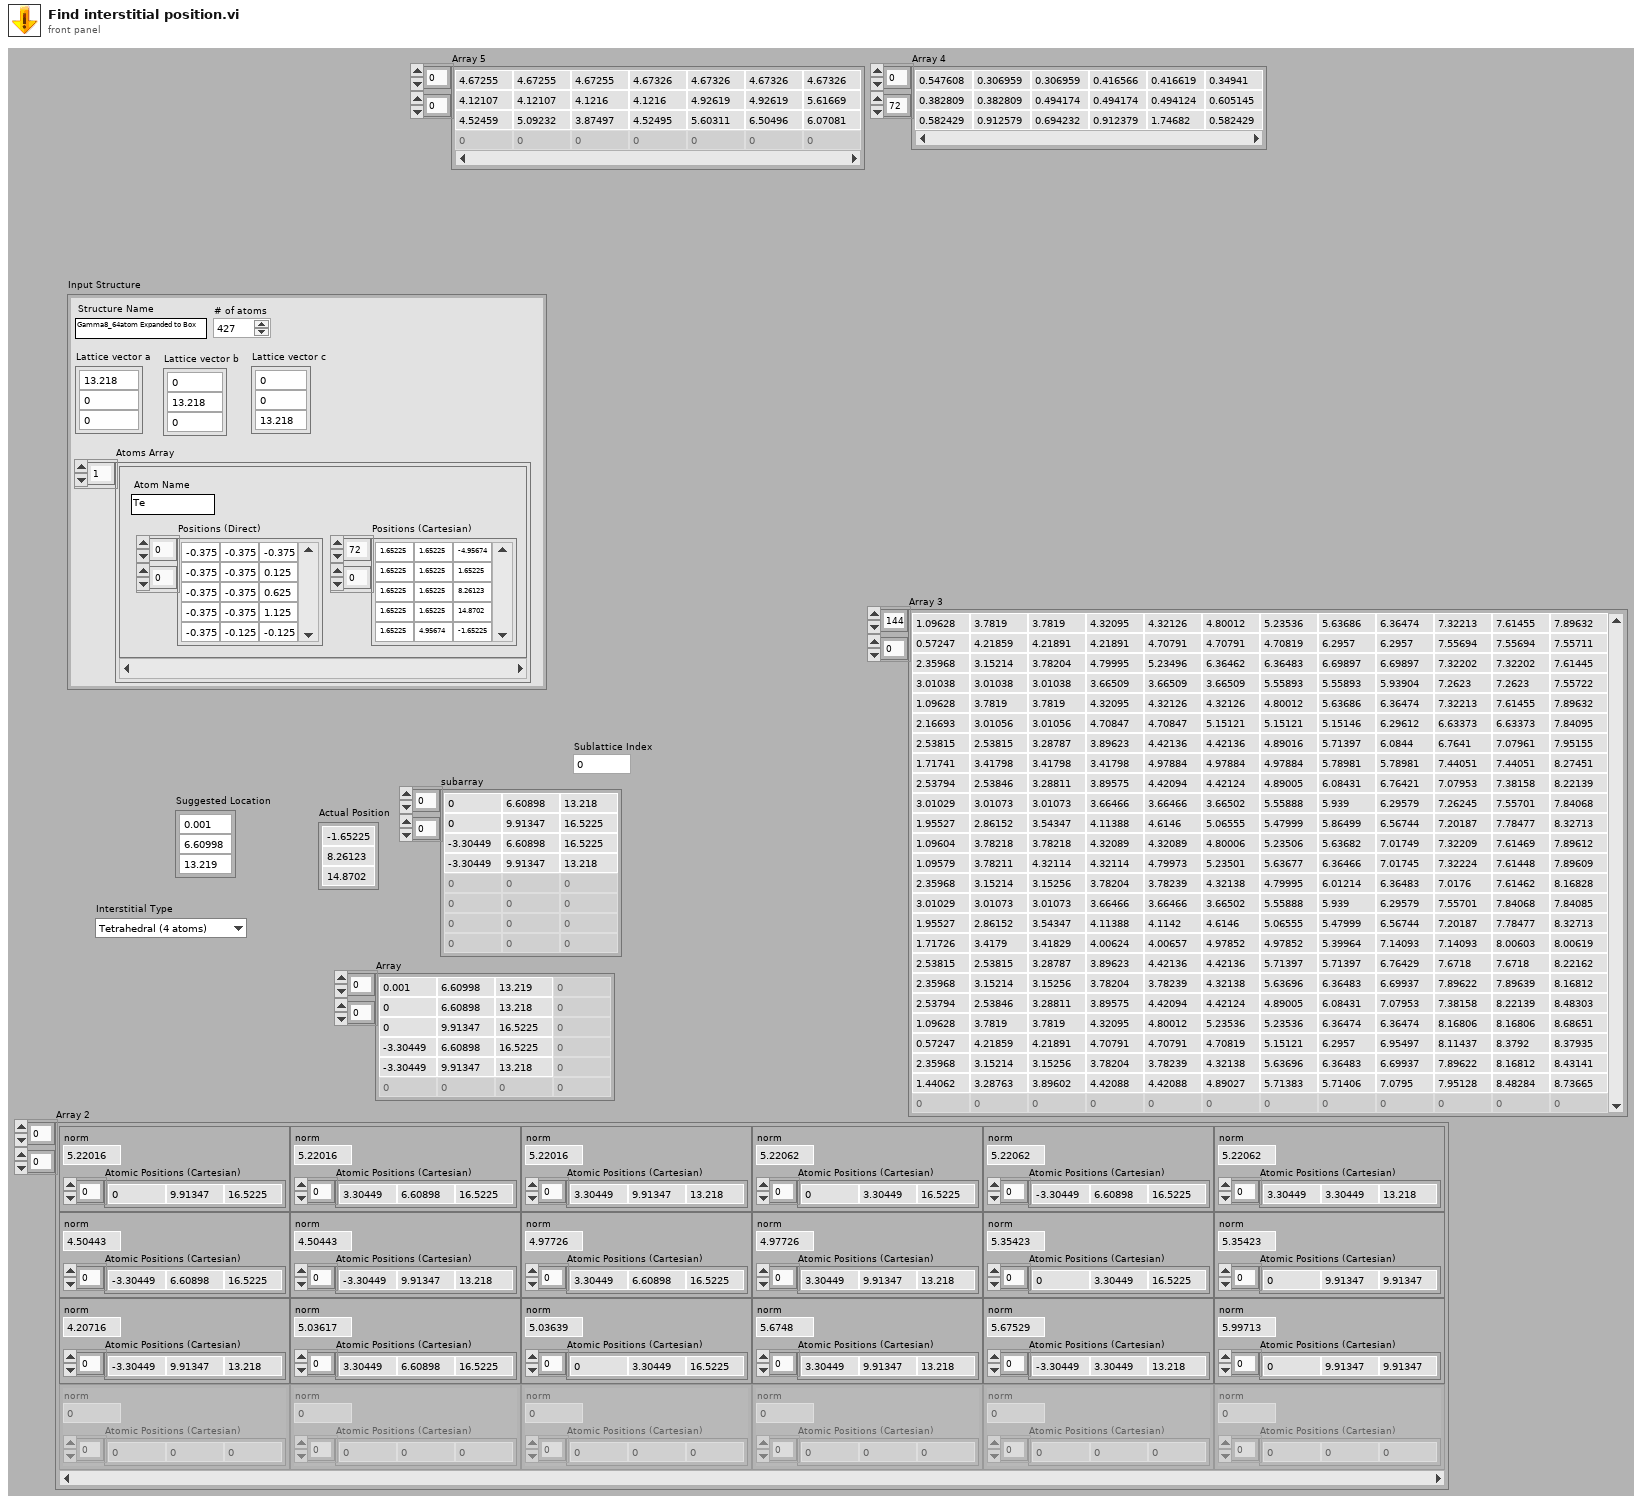
[diagram p1: front panel]
types:
  T1 = cluster{"Structure Name":string, "Lattice vector a":dbl[], "Lattice vector b":dbl[], "Lattice vector c":dbl[], "Atoms Array":cluster{"Atom Name":string, "Positions (Direct)":dbl[][], "Positions (Cartesian)":dbl[][]}[], "# of atoms":i32}
  T2 = cluster{"norm":dbl, "Atomic Positions (Cartesian)":dbl[]}[][]
  T3 = enum16{"Tetrahedral (4 atoms)", "Octahedral (6 atoms)"}
  T4 = cluster{"Atom Name":string, "Positions (Direct)":dbl[][], "Positions (Cartesian)":dbl[][]}[]
  T5 = cluster{"Atom Name":string, "Positions (Direct)":dbl[][], "Positions (Cartesian)":dbl[][]}
  T6 = cluster{"norm":dbl, "Positions (Cartesian)":dbl[]}
  T7 = cluster{"norm":dbl, "Positions (Cartesian)":dbl[]}[]
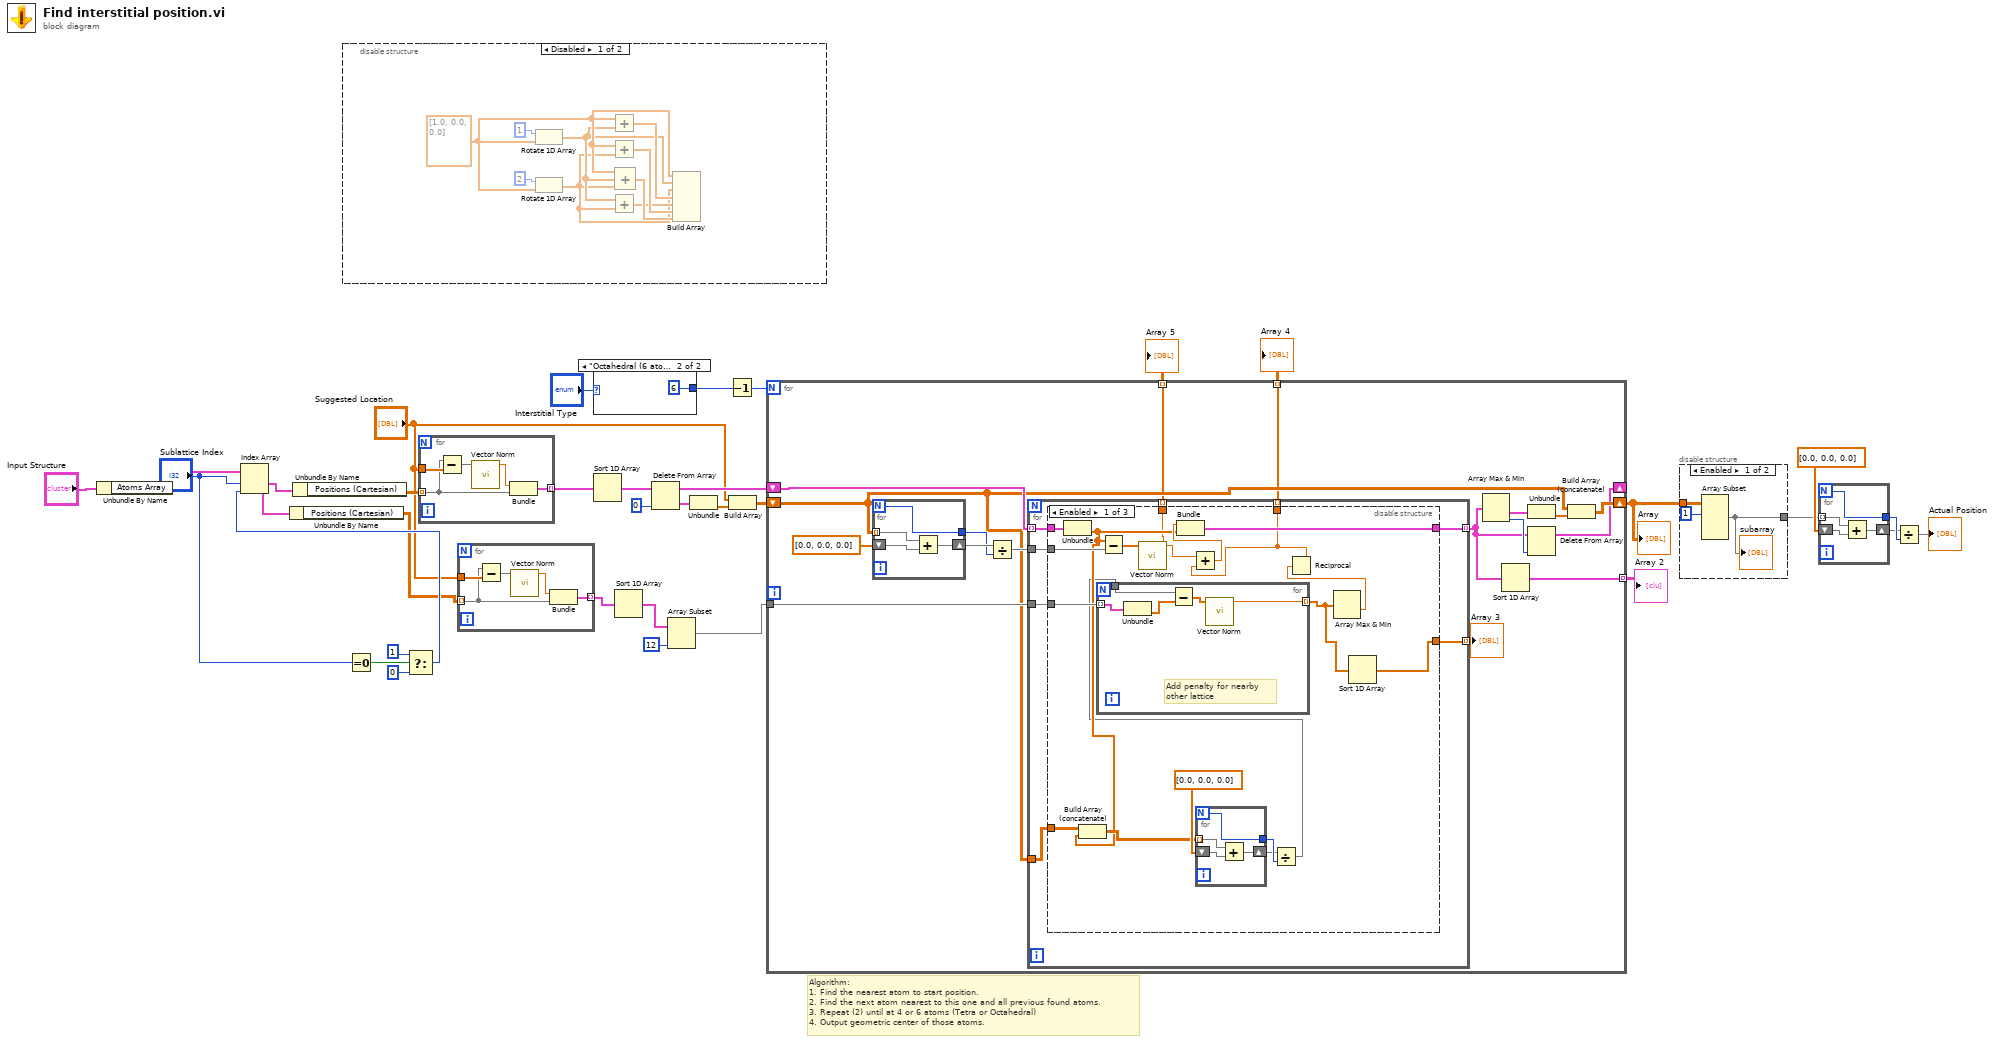
[diagram p0: block diagram]
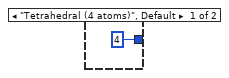
[diagram p4: hidden frame]
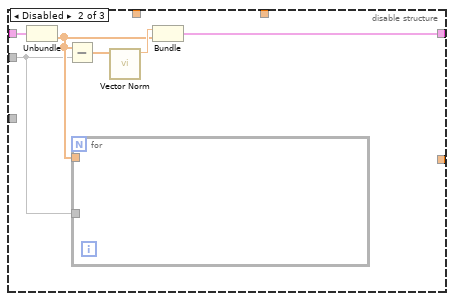
[diagram p5: hidden frame]
diagram:
  # "Algorithm:\n1. Find the nearest atom to start position.\n2. Find the next atom nearest to this one and all previous found atoms.\n3. Repeat (2) until at 4 or 6 atoms (Tetra or Octahedral)\n4. Output geometric center of those atoms."
  n1 = Unbundle By Name("Input Structure") -> ("Atoms Array"=w18:T4)
  n2 = disable-structure shown="Disabled" {
    frame Disabled {
      w40 = dbl[] [1.0, 0.0, 0.0]
      n3 = Rotate 1D Array(1:w40, 2:1 ("n")) -> (0:w39:dbl[])
      n4 = Rotate 1D Array(1:w40, 2:2 ("n")) -> (0:w38:dbl[])
      n5 = Add(x=w40, y=w39) -> (x+y=w41:dbl[])
      n6 = Add(x=w40, y=w38) -> (x+y=w43:dbl[])
      n7 = Add(x=w39, y=w38) -> (x+y=w42:dbl[])
      n8 = Compound Arithmetic op=unknown(w40, w39, w38) -> (w44:dbl[])
      n9 = Build Array(w40, w39, w38, w41, w42, w43, w44) -> ()  [unwired: 1 out]
    }
    frame Enabled {
    }
  }
  n10 = Equal To 0?(x="Sublattice Index") -> (x = 0?=w15:bool)
  n11 = Select(t=1, s=w15, f=0) -> (s? t:f=w12:i32)
  n12 = Index Array(array=w18, index #1="Sublattice Index", index #2=w12) -> (element #1=w17:T5, element #2=w11:T5)
  n13 = Unbundle By Name(w11) -> ("Positions (Cartesian)"=w10:dbl[][])
  n14 = Unbundle By Name(w17) -> ("Positions (Cartesian)"=w16:dbl[][])
  n15 = for {
    tunnel: w16 -> [w46] mode=indexing
    tunnel: "Suggested Location" -> [w49]
    tunnel: [w45] -> w33 mode=indexing
    n16 = Subtract(x=w46, y=w49) -> (x-y=w48:dbl[])
    n17 = call-poly <vilib>:"Vector Norm.vi"("Input Vector"=w48) -> ("norm"=w47:dbl)  [unwired: 9 in, 1 out]
    n18 = Bundle("norm"=w47, "Positions (Cartesian)"=w46) -> (w45:T6)  [unwired: 1 in]
  }
  n19 = for {
    tunnel: w10 -> [w51] mode=indexing
    tunnel: "Suggested Location" -> [w54]
    tunnel: [w50] -> w7 mode=indexing
    n20 = Subtract(x=w51, y=w54) -> (x-y=w53:dbl[])
    n21 = call-poly <vilib>:"Vector Norm.vi"("Input Vector"=w53) -> ("norm"=w52:dbl)  [unwired: 9 in, 1 out]
    n22 = Bundle("norm"=w52, "Positions (Cartesian)"=w51) -> (w50:T6)  [unwired: 1 in]
  }
  n23 = case shown="\"Octahedral (6 atoms)\"" "Interstitial Type" {
    tunnel: [4 6] -> w24
    frame "Tetrahedral (4 atoms)", Default {
    }
    frame "Octahedral (6 atoms)" {
    }
  }
  n24 = Sort 1D Array(array=w33) -> (sorted array=w8:T7)
  n25 = Sort 1D Array(array=w7) -> (sorted array=w6:T7)
  n26 = Delete From Array(array=w8, index=0) -> (deleted portion=w27:T6, array with subset deleted=w26:T7)  [unwired: 1 in]
  n27 = Array Subset(array=w6, length=12) -> (w4:T7)  [unwired: 1 in]
  n28 = Unbundle(w27) -> ("Positions (Cartesian)"=w34:dbl[])  [unwired: 1 out]
  n29 = Decrement(x=w24) -> (x-1=w23:i32)
  n30 = Build Array("Suggested Location", w34) -> (w35:dbl[][])
  n31 = for {
    N: w23 -> [_]
    shift-right: [w67] -> w22
    shift-left: w35 -> [w59]
    shift-right: [w64] -> _
    shift-left: w26 -> [w73]
    tunnel: [w62] -> w20 mode=indexing
    tunnel: w4 -> [w61]
    tunnel: [w58] -> w2 mode=indexing
    tunnel: [w57] -> w1 mode=indexing
    n32 = for {
      N -> [w74]
      tunnel: w59 -> [w77] mode=indexing
      shift-right: [w76] -> w71
      shift-left: dbl[] [0.0, 0.0, 0.0] -> [w75]
      tunnel: [w74] -> w70
      n33 = Add(x=w77, y=w75) -> (x+y=w76:dbl[])
    }
    n34 = Divide(x=w71, y=w70) -> (x/y=w66:dbl[])
    n35 = for {
      tunnel: w73 -> [w85] mode=indexing
      tunnel: w66 -> [w84]
      tunnel: [w83] -> w63 mode=indexing
      tunnel: w61 -> [w82]
      tunnel: [w81] -> w60 mode=indexing
      tunnel: w59 -> [w80]
      tunnel: [w79] -> w58 mode=indexing
      tunnel: [w78] -> w57 mode=indexing
      n36 = disable-structure shown="Enabled" {
        disable-tunnel: w85 -> [w103 w118 _]
        disable-tunnel: w84 -> [w101 w113 _]
        disable-tunnel: [w100 w115 _] -> w83
        disable-tunnel: w82 -> [w99 _ _]
        disable-tunnel: [w96 _ _] -> w81
        disable-tunnel: w80 -> [w90 _ _]
        disable-tunnel: [w87 _ _] -> w79
        disable-tunnel: [w86 _ _] -> w78
        frame Enabled {
          n37 = Unbundle(w103) -> ("Positions (Cartesian)"=w89:dbl[])  [unwired: 1 out]
          n38 = Build Array (concatenate)(w90, w89) -> (w91:dbl[][])
          n39 = Subtract(x=w89, y=w101) -> (x-y=w102:dbl[])
          n40 = call-poly <vilib>:"Vector Norm.vi"("Input Vector"=w102) -> ("norm"=w86:dbl)  [unwired: 9 in, 1 out]
          n41 = for {
            N -> [w104]
            tunnel: w91 -> [w107] mode=indexing
            shift-right: [w106] -> w93
            shift-left: dbl[] [0.0, 0.0, 0.0] -> [w105]
            tunnel: [w104] -> w94
            n42 = Add(x=w107, y=w105) -> (x+y=w106:dbl[])
          }
          n43 = Divide(x=w93, y=w94) -> (x/y=w88:dbl[])
          n44 = for {
            tunnel: w99 -> [w112] mode=indexing
            tunnel: w88 -> [w111]
            tunnel: [w108] -> w97 mode=indexing
            # "Add penalty for nearby \nother lattice"
            n45 = Unbundle(w112) -> ("Positions (Cartesian)"=w110:dbl[])  [unwired: 1 out]
            n46 = Subtract(x=w111, y=w110) -> (x-y=w109:dbl[])
            n47 = call-poly <vilib>:"Vector Norm.vi"("Input Vector"=w109) -> ("norm"=w108:dbl)  [unwired: 9 in, 1 out]
          }
          n48 = Array Max & Min(array=w97) -> (min value=w95:dbl)  [unwired: 3 out]
          n49 = Reciprocal(x=w95) -> (1/x=w87:dbl)
          n50 = Add(x=w86, y=w87) -> (x+y=w98:dbl)
          n51 = Bundle(w98, "Positions (Cartesian)"=w89) -> (w100:cluster{dbl, "Positions (Cartesian)":dbl[]})  [unwired: 1 in]
          n52 = Sort 1D Array(array=w97) -> (sorted array=w96:dbl[])
        }
        frame Disabled {
          n53 = Unbundle(w118) -> ("Positions (Cartesian)"=w114:dbl[])  [unwired: 1 out]
          n54 = Subtract(x=w114, y=w113) -> (x-y=w117:dbl[])
          n55 = for {
            tunnel: w114 -> [_]
            tunnel: w113 -> [_]
          }
          n56 = call-poly <vilib>:"Vector Norm.vi"("Input Vector"=w117) -> ("norm"=w116:dbl)  [unwired: 9 in, 1 out]
          n57 = Bundle("norm"=w116, "Positions (Cartesian)"=w114) -> (w115:T6)  [unwired: 1 in]
        }
        frame Disabled {
        }
      }
    }
    "Array 3" <- w60
    n58 = Array Max & Min(array=w63) -> (min value=w69:cluster{dbl, "Positions (Cartesian)":dbl[]}, min index (indices)=w65:i32)  [unwired: 2 out]
    n59 = Sort 1D Array(array=w63) -> (sorted array=w62:cluster{dbl, "Positions (Cartesian)":dbl[]}[])
    n60 = Unbundle(w69) -> ("Positions (Cartesian)"=w68:dbl[])  [unwired: 1 out]
    n61 = Delete From Array(array=w63, index=w65) -> (array with subset deleted=w64:cluster{dbl, "Positions (Cartesian)":dbl[]}[])  [unwired: 1 in, 1 out]
    n62 = Build Array (concatenate)(w59, w68) -> (w67:dbl[][])
  }
  "Array" <- w22
  "Array 2" <- w20
  "Array 4" <- w2
  "Array 5" <- w1
  n63 = disable-structure shown="Enabled" {
    disable-tunnel: w22 -> [w121 w122]
    disable-tunnel: [w119 w122] -> w21
    frame Enabled {
      n64 = Array Subset(array=w121, index (row)=1 ("index")) -> (w119:dbl[][])  [unwired: 3 in]
      "subarray" <- w119
    }
    frame Disabled {
    }
  }
  n65 = for {
    N -> [w123]
    tunnel: w21 -> [w126] mode=indexing
    shift-right: [w125] -> w31
    shift-left: dbl[] [0.0, 0.0, 0.0] -> [w124]
    tunnel: [w123] -> w32
    n66 = Add(x=w126, y=w124) -> (x+y=w125:dbl[])
  }
  n67 = Divide(x=w31, y=w32) -> (x/y=→"Actual Position":dbl[])
